vi "LPT-GUI-MIC-ver 5F 2.0.vi"() -> ()   [LabVIEW 2019]
uses:
  <vilib>/userDefined/High Color/IMAQdx.ctl
  LPT/LabView - DISB Eval SW 2.6/LabView - DISB Eval SW 2.6/Register name.ctl
  LPT/LPT-GUI-MIC-ver 5c GLOBAL 1.0.vi
  <vilib>/Utility/file.llb/Write Delimited Spreadsheet (DBL).vi
  <vilib>/vision/driver/NI_Vision_Acquisition_Software.lvlib
panel:
  out "Numeric 9":dbl
  out "Numeric 8":i32
  out "Numeric 7":i32
  out "Numeric 6":i32
  out "Numeric 5":i32
  out "Numeric 4":i32
  out "Numeric 3":i32
  out "Numeric 2":i32
  out "Numeric":i32
  in  "SHUTDOWN\nPROGRAM":bool
  in  "LASER\nOFF":bool
  out "EPOS 1":string
  in  "ACT":refnum<visa-resource-name>="COM5"
  in  "RAMAN Spectometer\n Parameters":T1={"Integration Time (ms)"=80, "Digitizer Clock Rate Setting"=3, "Number of Scans to Average"=1, "Optical Smoothing Level"=0, "C1"=0.096038248763, "C2"=3.43035e-07, "C3"=536.3, "C4"=-1.607e-09, 12}
  in  "LED":refnum<visa-resource-name>="COM5"
  in  "Session In 2":T2="cam6"
  in  "Session In":T2="cam5"
  out "COMMAND1 READ 3":string="LED1 ON\r"
  out "AUT FOCUS STATUS 2":bool
  out "Position (um) 2":dbl(slide) min=0.0 max=100.0 step=0.01 scale=0.0..1500.0
  out "COMMAND 3":string="LED1 OFF"
  out "NUMBER 2":string
  out "Raw Data 2":sgl[](graph)
  out "power sum 2":sgl
  in  "#of steps 3":i32=200
  in  "STAGE START 2":i32
  in  "STAGE STOP 2":i32=20
  out "power sum":sgl
  out "Raw Data":sgl[](graph)
  in  "START CAM TAB":bool
  out "Camera STOP 2":bool
  out "COMMAND1 READ 2":string="LED1 ON\r"
  out "Position (um)":dbl(slide)=1400.0 min=0.0 max=100.0 step=0.01 scale=-10000.0..10000.0
  out "COMMAND 2":string="LED1 OFF"
  out "NUMBER":string
  in  "#of steps 2":i32=5
  in  "STAGE START":i32=-10000
  in  "STAGE STOP":i32=10000
  out "BOROSCOPE END":string
  out "Position (mm)":dbl(slide)=10.0 min=0.0 max=100.0 step=0.01 scale=0.0..20.0 scale format="%.2f"
  out "COMMAND1 READ":string="LED1 ON\r"
  in  "COMMAND 1":string="LED1 OFF"
  out "LASER \nFOCUSED":bool
  in  "INTERACTIVE CONTROLS":T3(radio)
  in  "LQC":refnum<visa-resource-name>="COM4" caption="LQComm resource name"
  in  "ANALYSIS PROGRAM":T4(radio)
  in  "LIBS Laser Frequency (Hz)":u16=10 min=10 max=1000
  in  "Auto Set\nLaser Frequency":bool
  in  "AQUISITION TYPE":enum32{"RAMAN", "LIBS"}(radio)
  in  "Integration\n Time (ms)":i32=100
  in  "ID SPECTRA":bool
  in  "Number of Scans  to Acquire":i32=2
  in  "AutoAcquire":bool=TRUE
  out "power setting from LQ":string="POWER=080\r\n"
  out "Power Out":dbl=0.4
  in  "Get Dark?":bool
  in  "Set Power (mW)":i32=80
  in  "Start":bool
  in  "CAMERA STOP":bool
  in  "EXIT INTERACTIVE\nCONTROL":bool
  in  "ABORT \nLOOP":bool
  out "Removed background":dbl[](graph)
  out "LIBS Dark Spectra":dbl[](graph)
  out "Dark Spectra":dbl[](graph)=[1870.0, 1885.0, 1880.0, 1896.0, 1901.0, 1906.0, 1893.0, 1873.0, 1869.0, 1877.0, 1867.0, 1828.0, 1817.0, 1812.0, 1819.0, 1837.0, 1828.0, 1798.0, 1797.0, 1809.0, 1800.0, 1781.0, 1773.0, 1752.0, 1749.0, 1759.0, 1771.0, 1780.0, 1783.0, 1757.0, 1759.0, 1773.0, 1764.0, 1750.0, 1783.0, 1813.0, 1852.0, 1868.0, 1849.0, 1845.0, 1844.0, 1863.0, 1853.0, 1841.0, 1791.0, 1771.0, 1777.0, 1785.0, 1821.0, 1881.0, 1909.0, 1926.0, 1925.0, 1929.0, 1912.0, 1898.0, 1903.0, 1901.0, 1897.0, 1865.0, 1874.0, 1897.0, 1919.0, 1905.0, 1901.0, 1919.0, 1947.0, 1919.0, 1887.0, 1877.0, 1837.0, 1807.0, 1823.0, 1855.0, 1871.0, 1847.0, 1823.0, 1842.0, 1887.0, 1906.0, 1925.0, 1945.0, 1924.0, 1919.0, 1919.0, 1906.0, 1897.0, 1865.0, 1817.0, 1801.0, 1809.0, 1797.0, 1818.0, 1860.0, 1853.0, 1819.0, 1768.0, 1758.0, 1741.0, 1732.0, 1717.0, 1725.0, 1734.0, 1713.0, 1695.0, 1707.0, 1727.0, 1743.0, 1759.0, 1788.0, 1802.0, 1775.0, 1772.0, 1780.0, 1801.0, 1819.0, 1813.0, 1817.0, 1823.0, 1844.0, 1851.0, 1805.0, 1809.0, 1842.0, 1845.0, 1853.0, 1837.0, 1846.0, 1837.0, 1853.0, 1862.0, 1881.0, 1901.0, 1874.0, 1861.0, 1892.0, 1876.0, 1872.0, 1855.0, 1846.0, 1860.0, 1861.0, 1887.0, 1887.0, 1883.0, 1897.0, 1897.0, 1903.0, 1911.0, 1901.0, 1880.0, 1871.0, 1855.0, 1879.0, 1860.0, 1871.0, 1880.0, 1879.0, 1858.0, 1855.0, 1837.0, 1837.0, 1823.0, 1828.0, 1807.0, 1821.0, 1882.0, 1890.0, 1893.0, 1860.0, 1832.0, 1812.0, 1813.0, 1842.0, 1852.0, 1849.0, 1851.0, 1835.0, 1849.0, 1885.0, 1924.0, 1930.0, 1930.0, 1925.0, 1892.0, 1897.0, 1903.0, 1900.0, 1912.0, 1917.0, 1946.0, 1947.0, 1927.0, 1896.0, 1881.0, 1896.0, 1874.0, 1873.0, 1876.0, 1898.0, 1899.0, 1885.0, 1892.0, 1897.0, 1896.0, 1896.0, 1878.0, 1870.0, 1860.0, 1853.0, 1867.0, 1855.0, 1839.0, 1839.0, 1849.0, 1853.0, 1846.0, 1829.0, 1817.0, 1828.0, 1823.0, 1860.0, 1881.0, 1863.0, 1885.0, 1860.0, 1833.0, 1846.0, 1832.0, 1844.0, 1813.0, 1815.0, 1837.0, 1833.0, 1837.0, 1828.0, 1829.0, 1844.0, 1840.0, 1849.0, 1844.0, 1812.0, 1815.0, 1801.0, 1814.0, 1815.0, 1837.0, 1832.0, 1840.0, 1812.0, 1797.0, 1815.0, 1862.0, 1899.0, 1906.0, 1905.0, 1885.0, 1868.0, 1861.0, 1845.0, 1832.0, 1797.0, 1803.0, 1791.0, 1791.0, 1784.0, 1801.0, 1786.0, 1768.0, 1765.0, 1759.0, 1745.0, 1743.0, 1774.0, 1813.0, 1820.0, 1855.0, 1881.0, 1881.0, 1887.0, 1876.0, 1870.0, 1864.0, 1897.0, 1897.0, 1887.0, 1873.0, 1853.0, 1833.0, 1807.0, 1802.0, 1791.0, 1823.0, 1828.0, 1812.0, 1850.0, 1853.0, 1846.0, 1839.0, 1837.0, 1852.0, 1849.0, 1828.0, 1848.0, 1864.0, 1860.0, 1864.0, 1846.0, 1829.0, 1837.0, 1835.0, 1819.0, 1807.0, 1812.0, 1805.0, 1789.0, 1798.0, 1802.0, 1818.0, 1783.0, 1796.0, 1804.0, 1837.0, 1876.0, 1935.0, 1994.0, 2007.0, 1969.0, 1961.0, 1938.0, 1917.0, 1908.0, 1901.0, 1885.0, 1911.0, 1930.0, 1929.0, 1945.0, 1919.0, 1899.0, 1870.0, 1855.0, 1825.0, 1814.0, 1817.0, 1797.0, 1803.0, 1791.0, 1789.0, 1768.0, 1734.0, 1757.0, 1757.0, 1737.0, 1752.0, 1773.0, 1768.0, 1761.0, 1759.0, 1784.0, 1783.0, 1803.0, 1791.0, 1791.0, 1796.0, 1791.0, 1781.0, 1773.0, 1761.0, 1780.0, 1791.0, 1780.0, 1773.0, 1759.0, 1757.0, 1769.0, 1773.0, 1768.0, 1780.0, 1780.0, 1782.0, 1807.0, 1805.0, 1789.0, 1807.0, 1836.0, 1823.0, 1839.0, 1873.0, 1873.0, 1893.0, 1892.0, 1868.0, 1876.0, 1887.0, 1896.0, 1899.0, 1892.0, 1867.0, 1851.0, 1848.0, 1839.0, 1865.0, 1866.0, 1849.0, 1834.0, 1839.0, 1862.0, 1861.0, 1851.0, 1839.0, 1849.0, 1847.0, 1828.0, 1789.0, 1769.0, 1787.0, 1779.0, 1797.0, 1816.0, 1846.0, 1855.0, 1855.0, 1863.0, 1869.0, 1885.0, 1892.0, 1901.0, 1946.0, 1913.0, 1880.0, 1896.0, 1901.0, 1877.0, 1881.0, 1878.0, 1855.0, 1845.0, 1832.0, 1799.0, 1769.0, 1757.0, 1781.0, 1762.0, 1735.0, 1714.0, 1733.0, 1757.0, 1773.0, 1773.0, 1783.0, 1778.0, 1768.0, 1764.0, 1765.0, 1753.0, 1738.0, 1759.0, 1781.0, 1789.0, 1800.0, 1799.0, 1796.0, 1785.0, 1771.0, 1727.0, 1700.0, 1723.0, 1711.0, 1716.0, 1738.0, 1773.0, 1781.0, 1769.0, 1778.0, 1768.0, 1771.0, 1775.0, 1781.0, 1768.0, 1744.0, 1739.0, 1732.0, 1716.0, 1695.0, 1689.0, 1695.0, 1679.0, 1695.0, 1692.0, 1717.0, 1718.0, 1721.0, 1695.0, 1679.0, 1677.0, 1675.0, 1678.0, 1679.0, 1682.0, 1689.0, 1684.0, 1711.0, 1711.0, 1721.0, 1727.0, 1727.0, 1723.0, 1707.0, 1732.0, 1721.0, 1724.0, 1700.0, 1692.0, 1685.0, 1693.0, 1695.0, 1705.0, 1694.0, 1700.0, 1722.0, 1714.0, 1719.0, 1723.0, 1711.0, 1721.0, 1746.0, 1775.0, 1756.0, 1704.0, 1692.0, 1721.0, 1725.0, 1718.0, 1712.0, 1725.0, 1732.0, 1741.0, 1745.0, 1773.0, 1784.0, 1782.0, 1785.0, 1800.0, 1800.0, 1785.0, 1757.0, 1759.0, 1718.0, 1725.0, 1725.0, 1736.0, 1770.0, 1802.0, 1808.0, 1801.0, 1809.0, 1812.0, 1794.0, 1823.0, 1842.0, 1839.0, 1849.0, 1823.0, 1832.0, 1823.0, 1801.0, 1812.0, 1832.0, 1823.0, 1810.0, 1810.0, 1796.0, 1816.0, 1797.0, 1853.0, 1871.0, 1883.0, 1887.0, 1902.0, 1884.0, 1869.0, 1853.0, 1832.0, 1823.0, 1812.0, 1821.0, 1823.0, 1832.0, 1821.0, 1823.0, 1809.0, 1784.0, 1752.0, 1732.0, 1727.0, 1721.0, 1709.0, 1735.0, 1727.0, 1725.0, 1707.0, 1698.0, 1682.0, 1689.0, 1714.0, 1716.0, 1707.0, 1709.0, 1714.0, 1725.0, 1727.0, 1738.0, 1725.0, 1741.0, 1739.0, 1701.0, 1733.0, 1727.0, 1717.0, 1718.0, 1752.0, 1775.0, 1775.0, 1784.0, 1802.0, 1771.0, 1759.0, 1750.0, 1724.0, 1721.0, 1711.0, 1689.0, 1677.0, 1666.0, 1686.0, 1698.0, 1711.0, 1750.0, 1741.0, 1756.0, 1771.0, 1768.0, 1787.0, 1796.0, 1807.0, 1790.0, 1809.0, 1842.0, 1832.0, 1807.0, 1805.0, 1805.0, 1764.0, 1789.0, 1785.0, 1669.0, 1625.0, 1631.0, 1637.0, 1642.0, 1599.0, 1605.0, 1579.0, 1592.0, 1576.0, 1590.0, 1604.0, 1615.0, 1659.0, 1672.0, 1669.0, 1689.0, 1672.0, 1672.0, 1701.0, 1716.0, 1741.0, 1730.0, 1719.0, 1711.0, 1695.0, 1706.0, 1721.0, 1770.0, 1796.0, 1797.0, 1768.0, 1765.0, 1781.0, 1765.0, 1759.0, 1749.0, 1781.0, 1786.0, 1804.0, 1796.0, 1777.0, 1768.0, 1772.0, 1778.0, 1821.0, 1821.0, 1823.0, 1837.0, 1845.0, 1829.0, 1849.0, 1833.0, 1832.0, 1797.0, 1771.0, 1764.0, 1791.0, 1786.0, 1764.0, 1743.0, 1730.0, 1752.0, 1746.0, 1741.0, 1741.0, 1748.0, 1757.0, 1784.0, 1775.0, 1777.0, 1796.0, 1810.0, 1799.0, 1814.0, 1768.0, 1773.0, 1780.0, 1765.0, 1764.0, 1769.0, 1748.0, 1732.0, 1709.0, 1706.0, 1695.0, 1679.0, 1675.0, 1669.0, 1679.0, 1707.0, 1721.0, 1711.0, 1704.0, 1701.0, 1700.0, 1695.0, 1695.0, 1668.0, 1692.0, 1711.0, 1725.0, 1716.0, 1693.0, 1700.0, 1720.0, 1704.0, 1711.0, 1716.0, 1725.0, 1721.0, 1706.0, 1700.0, 1706.0, 1717.0, 1732.0, 1717.0, 1721.0, 1695.0, 1695.0, 1698.0, 1688.0, 1689.0, 1691.0, 1687.0, 1709.0, 1717.0, 1732.0, 1725.0, 1668.0, 1672.0, 1673.0, 1681.0, 1688.0, 1707.0, 1725.0, 1739.0, 1716.0, 1641.0, 1636.0, 1642.0, 1655.0, 1663.0, 1675.0, 1675.0, 1700.0, 1730.0, 1764.0, 1803.0, 1816.0, 1820.0, 1807.0, 1791.0, 1759.0, 1753.0, 1761.0, 1759.0, 1753.0, 1744.0, 1775.0, 1781.0, 1768.0, 1753.0, 1741.0, 1721.0, 1725.0, 1743.0, 1748.0, 1747.0, 1771.0, 1775.0, 1771.0, 1756.0, 1753.0, 1709.0, 1716.0, 1704.0, 1734.0, 1737.0, 1725.0, 1721.0, 1724.0, 1716.0, 1732.0, 1744.0, 1775.0, 1751.0, 1706.0, 1704.0, 1716.0, 1709.0, 1717.0, 1741.0, 1761.0, 1764.0, 1781.0, 1791.0, 1764.0, 1746.0, 1732.0, 1734.0, 1727.0, 1716.0, 1700.0, 1686.0, 1684.0, 1686.0, 1707.0, 1732.0, 1727.0, 1738.0, 1716.0, 1705.0, 1709.0, 1707.0, 1700.0, 1698.0, 1698.0, 1716.0, 1723.0, 1705.0, 1717.0, 1689.0, 1690.0, 1687.0, 1684.0, 1719.0, 1717.0, 1714.0, 1690.0, 1668.0, 1663.0, 1675.0, 1677.0, 1684.0, 1673.0, 1668.0, 1679.0, 1695.0, 1706.0, 1735.0, 1748.0, 1747.0, 1759.0, 1764.0, 1757.0, 1732.0, 1750.0, 1781.0, 1764.0, 1764.0, 1749.0, 1754.0, 1756.0, 1741.0, 1739.0, 1741.0, 1714.0, 1733.0, 1762.0, 1759.0, 1768.0, 1775.0, 1768.0, 1759.0, 1768.0, 1750.0, 1739.0, 1757.0, 1757.0, 1727.0, 1748.0, 1723.0, 1725.0, 1709.0, 1709.0, 1709.0, 1731.0, 1734.0, 1748.0, 1759.0, 1757.0, 1759.0, 1752.0, 1741.0, 1755.0, 1787.0, 1791.0, 1820.0, 1840.0, 1860.0, 1873.0, 1874.0, 1865.0, 1876.0, 1876.0, 1844.0, 1844.0, 1849.0, 1862.0, 1832.0, 1828.0, 1842.0, 1832.0, 1796.0, 1788.0, 1751.0, 1764.0, 1756.0, 1746.0, 1739.0, 1733.0, 1726.0, 1705.0, 1700.0, 1723.0, 1725.0, 1725.0, 1739.0, 1759.0, 1777.0, 1771.0, 1759.0, 1771.0, 1765.0, 1753.0, 1725.0, 1684.0, 1647.0, 1636.0, 1652.0, 1657.0, 1669.0, 1672.0, 1677.0, 1653.0, 1672.0, 1657.0, 1661.0, 1660.0, 1676.0, 1704.0, 1707.0, 1729.0, 1757.0, 1796.0, 1797.0, 1802.0, 1797.0, 1807.0, 1844.0, 1835.0, 1794.0, 1791.0, 1796.0, 1801.0, 1789.0, 1791.0, 1782.0, 1768.0, 1739.0, 1723.0, 1736.0, 1732.0, 1737.0, 1733.0, 1727.0, 1707.0, 1677.0, 1695.0, 1704.0, 1714.0, 1690.0, 1657.0, 1661.0, 1669.0, 1656.0, 1652.0, 1611.0, 1595.0, 1549.0, 1562.0, 1596.0, 1610.0, 1573.0, 1576.0, 1577.0, 1567.0, 1573.0, 1605.0, 1592.0, 1622.0, 1621.0, 1609.0, 1599.0, 1606.0, 1581.0, 1565.0, 1567.0, 1589.0, 1610.0, 1607.0, 1608.0, 1643.0, 1647.0, 1668.0, 1691.0, 1675.0, 1641.0, 1647.0, 1640.0, 1622.0, 1621.0, 1588.0, 1602.0, 1622.0, 1611.0, 1599.0, 1602.0, 1640.0, 1643.0, 1647.0, 1629.0, 1577.0, 1547.0, 1554.0, 1551.0, 1540.0, 1561.0, 1561.0, 1576.0, 1614.0, 1674.0, 1707.0, 1717.0, 1736.0, 1735.0, 1743.0, 1738.0, 1727.0, 1735.0, 1721.0, 1721.0, 1687.0, 1707.0, 1709.0, 1748.0, 1743.0, 1743.0, 1753.0, 1769.0, 1759.0, 1765.0, 1737.0, 1727.0, 1711.0, 1679.0, 1672.0, 1686.0, 1672.0, 1668.0, 1660.0, 1645.0, 1669.0, 1688.0, 1685.0, 1679.0, 1721.0, 1739.0, 1712.0, 1681.0, 1650.0, 1653.0, 1661.0, 1663.0, 1663.0, 1668.0, 1672.0, 1704.0, 1714.0, 1721.0, 1718.0, 1814.0, 1797.0, 1759.0, 1754.0, 1743.0, 1762.0, 1748.0, 1768.0, 1741.0, 1690.0, 1707.0, 1717.0, 1739.0, 1768.0, 1727.0, 1682.0, 1650.0, 1681.0, 1701.0, 1727.0, 1695.0, 1676.0, 1673.0, 1669.0, 1677.0, 1663.0, 1674.0, 1690.0, 1687.0, 1668.0, 1690.0, 1725.0, 1689.0, 1647.0, 1627.0, 1615.0, 1647.0, 1656.0, 1631.0, 1625.0, 1618.0, 1609.0, 1608.0, 1636.0, 1674.0, 1720.0, 1738.0, 1745.0, 1736.0, 1738.0, 1762.0, 1781.0, 1776.0, 1794.0, 1798.0, 1757.0, 1741.0, 1717.0, 1711.0, 1725.0, 1727.0, 1732.0, 1730.0, 1701.0, 1700.0, 1657.0, 1652.0, 1668.0, 1653.0, 1621.0, 1629.0, 1611.0, 1615.0, 1608.0, 1583.0, 1599.0, 1636.0, 1668.0, 1684.0, 1705.0, 1701.0, 1725.0, 1752.0, 1746.0, 1749.0, 1727.0, 1755.0, 1746.0, 1749.0, 1764.0, 1752.0, 1739.0, 1768.0, 1757.0, 1711.0, 1677.0, 1657.0, 1653.0, 1661.0, 1647.0, 1618.0, 1620.0, 1649.0, 1675.0, 1668.0, 1672.0, 1679.0, 1656.0, 1669.0, 1674.0, 1700.0, 1705.0, 1704.0, 1700.0, 1705.0, 1718.0, 1711.0, 1705.0, 1701.0, 1718.0, 1713.0, 1736.0, 1752.0, 1748.0, 1732.0, 1750.0, 1765.0, 1741.0, 1723.0, 1725.0, 1705.0, 1676.0, 1641.0, 1636.0, 1631.0, 1631.0, 1656.0, 1663.0, 1666.0, 1668.0, 1669.0, 1629.0, 1647.0, 1610.0, 1551.0, 1494.0, 1483.0, 1465.0, 1476.0, 1487.0, 1512.0, 1553.0, 1573.0, 1556.0, 1501.0, 1503.0, 1531.0, 1567.0, 1624.0, 1663.0, 1661.0, 1657.0, 1645.0, 1616.0, 1621.0, 1594.0, 1529.0, 1503.0, 1490.0, 1476.0, 1501.0, 1501.0, 1517.0, 1527.0, 1558.0, 1567.0, 1586.0, 1556.0, 1547.0, 1548.0, 1551.0, 1497.0, 1439.0, 1428.0, 1459.0, 1516.0, 1563.0, 1558.0, 1609.0, 1657.0, 1693.0, 1734.0, 1753.0, 1765.0, 1773.0, 1796.0, 1800.0, 1815.0, 1821.0, 1851.0, 1855.0, 1844.0, 1844.0, 1846.0, 1850.0, 1833.0, 1786.0, 1791.0, 1791.0, 1789.0, 1798.0, 1797.0, 1802.0, 1809.0, 1819.0, 1820.0, 1816.0, 1796.0, 1804.0, 1804.0, 1786.0, 1794.0, 1753.0, 1764.0, 1800.0, 1811.0, 1809.0, 1816.0, 1785.0, 1765.0, 1735.0, 1687.0, 1672.0, 1661.0, 1621.0, 1583.0, 1482.0, 1444.0, 1451.0, 1471.0, 1500.0, 1541.0, 1530.0, 1541.0, 1540.0, 1581.0, 1605.0, 1649.0, 1659.0, 1660.0, 1654.0, 1672.0, 1668.0, 1691.0, 1692.0, 1693.0, 1672.0, 1674.0, 1693.0, 1707.0, 1735.0, 1759.0, 1758.0, 1752.0, 1759.0, 1763.0, 1764.0, 1757.0, 1741.0, 1727.0, 1727.0, 1720.0, 1738.0, 1733.0, 1735.0, 1725.0, 1743.0, 1746.0, 1753.0, 1752.0, 1750.0, 1738.0, 1755.0, 1746.0, 1764.0, 1787.0, 1775.0, 1748.0, 1725.0, 1725.0, 1759.0, 1775.0, 1791.0, 1804.0, 1823.0, 1842.0, 1839.0, 1846.0, 1807.0, 1812.0, 1835.0, 1819.0, 1837.0, 1799.0, 1769.0, 1765.0, 1759.0, 1781.0, 1768.0, 1727.0, 1689.0, 1672.0, 1636.0, 1629.0, 1629.0, 1647.0, 1645.0, 1641.0, 1640.0, 1658.0, 1640.0, 1642.0, 1645.0, 1672.0, 1700.0, 1701.0, 1688.0, 1709.0, 1727.0, 1732.0, 1759.0, 1754.0, 1765.0, 1746.0, 1727.0, 1725.0, 1759.0, 1752.0, 1753.0, 1768.0, 1759.0, 1764.0, 1759.0, 1773.0, 1794.0, 1796.0, 1791.0, 1812.0, 1805.0, 1810.0, 1801.0, 1791.0, 1782.0, 1787.0, 1775.0, 1775.0, 1775.0, 1780.0, 1783.0, 1807.0, 1815.0, 1821.0, 1800.0, 1823.0, 1819.0, 1801.0, 1779.0, 1773.0, 1780.0, 1788.0, 1804.0, 1800.0, 1789.0, 1757.0, 1743.0, 1727.0, 1721.0, 1732.0, 1720.0, 1681.0, 1681.0, 1701.0, 1684.0, 1650.0, 1645.0, 1656.0, 1684.0, 1686.0, 1677.0, 1691.0, 1685.0, 1700.0, 1721.0, 1741.0, 1758.0, 1749.0, 1733.0, 1695.0, 1701.0, 1687.0, 1712.0, 1721.0, 1738.0, 1759.0, 1796.0, 1823.0, 1849.0, 1860.0, 1868.0, 1855.0, 1848.0, 1855.0, 1844.0, 1809.0, 1810.0, 1832.0, 1807.0, 1800.0, 1829.0, 1837.0, 1823.0, 1805.0, 1828.0, 1848.0, 1855.0, 1838.0, 1807.0, 1804.0, 1802.0, 1806.0, 1823.0, 1807.0, 1807.0, 1816.0, 1844.0, 1862.0, 1879.0, 1882.0, 1877.0, 1875.0, 1897.0, 1855.0, 1837.0, 1835.0, 1817.0, 1810.0, 1789.0, 1751.0, 1741.0, 1723.0, 1722.0, 1718.0, 1752.0, 1773.0, 1768.0, 1781.0, 1739.0, 1709.0, 1693.0, 1709.0, 1722.0, 1727.0, 1724.0, 1749.0, 1725.0, 1748.0, 1758.0, 1769.0, 1778.0, 1771.0, 1770.0, 1745.0, 1736.0, 1771.0, 1768.0, 1748.0, 1756.0, 1773.0, 1748.0, 1754.0, 1772.0, 1804.0, 1803.0, 1805.0, 1768.0, 1750.0, 1764.0, 1741.0, 1748.0, 1727.0, 1707.0, 1707.0, 1737.0, 1721.0, 1717.0, 1722.0, 1720.0, 1734.0, 1750.0, 1725.0, 1725.0, 1736.0, 1691.0, 1681.0, 1689.0, 1677.0, 1675.0, 1707.0, 1712.0, 1704.0, 1684.0, 1679.0, 1677.0, 1683.0, 1663.0, 1636.0, 1640.0, 1640.0, 1657.0, 1669.0, 1677.0, 1704.0, 1727.0, 1769.0, 1741.0, 1749.0, 1759.0, 1757.0, 1762.0, 1750.0, 1749.0, 1759.0, 1759.0, 1775.0, 1773.0, 1823.0, 1815.0, 1807.0, 1821.0, 1813.0, 1805.0, 1817.0, 1813.0, 1821.0, 1807.0, 1803.0, 1805.0, 1821.0, 1828.0, 1817.0, 1805.0, 1802.0, 1791.0, 1776.0, 1768.0, 1770.0, 1755.0, 1738.0, 1764.0, 1757.0, 1751.0, 1759.0, 1762.0, 1786.0, 1771.0, 1775.0, 1801.0, 1807.0, 1797.0, 1786.0, 1855.0, 1879.0, 1878.0, 1852.0, 1834.0, 1845.0, 1849.0, 1869.0, 1865.0, 1855.0, 1885.0, 1885.0, 1860.0, 1812.0, 1803.0, 1790.0, 1784.0, 1773.0, 1769.0, 1751.0, 1739.0, 1721.0, 1749.0, 1738.0, 1742.0, 1743.0, 1718.0, 1687.0, 1685.0, 1700.0, 1724.0, 1753.0, 1746.0, 1745.0, 1781.0, 1810.0, 1812.0, 1823.0, 1805.0, 1821.0, 1820.0, 1790.0, 1780.0, 1791.0, 1798.0, 1804.0, 1837.0, 1869.0, 1871.0, 1884.0, 1887.0, 1887.0, 1906.0, 1906.0, 1917.0, 1897.0, 1870.0, 1892.0, 1885.0, 1866.0, 1855.0, 1861.0, 1840.0, 1849.0, 1860.0, 1853.0, 1823.0, 1832.0, 1855.0, 1853.0, 1853.0, 1836.0, 1832.0, 1829.0, 1835.0, 1819.0, 1805.0, 1797.0, 1770.0, 1768.0, 1769.0, 1796.0, 1759.0, 1766.0, 1780.0, 1822.0, 1839.0, 1876.0, 1892.0, 1878.0, 1865.0, 1846.0, 1844.0, 1817.0, 1828.0, 1821.0, 1807.0, 1801.0, 1771.0, 1807.0, 1783.0, 1789.0, 1778.0, 1787.0, 1780.0, 1765.0, 1768.0, 1773.0, 1777.0, 1773.0, 1775.0, 1781.0, 1771.0, 1777.0, 1789.0, 1802.0, 1818.0, 1823.0, 1805.0, 1804.0, 1801.0, 1802.0, 1828.0, 1791.0, 1784.0, 1765.0, 1756.0, 1748.0, 1727.0, 1712.0, 1714.0, 1749.0, 1775.0, 1789.0, 1780.0, 1781.0, 1756.0, 1755.0, 1759.0, 1771.0, 1759.0, 1755.0, 1748.0, 1748.0, 1743.0, 1708.0, 1707.0, 1704.0, 1672.0, 1650.0, 1631.0, 1650.0, 1652.0, 1652.0, 1660.0, 1669.0, 1685.0, 1713.0, 1711.0, 1692.0, 1734.0, 1753.0, 1753.0, 1759.0, 1727.0, 1736.0, 1771.0, 1786.0, 1789.0, 1764.0, 1732.0, 1736.0, 1737.0, 1736.0, 1736.0, 1761.0, 1768.0, 1759.0, 1768.0, 1748.0, 1716.0, 1723.0, 1733.0, 1725.0, 1727.0, 1738.0, 1727.0, 1732.0, 1735.0, 1756.0, 1791.0, 1791.0, 1796.0, 1832.0, 1865.0, 1885.0, 1884.0, 1885.0, 1873.0, 1878.0, 1855.0, 1821.0, 1812.0, 1819.0, 1823.0, 1809.0, 1816.0, 1813.0, 1808.0, 1803.0, 1807.0, 1795.0, 1805.0, 1823.0, 1821.0, 1839.0, 1844.0, 1861.0, 1861.0, 1892.0, 1913.0, 1919.0, 1885.0, 1885.0, 1885.0, 1869.0, 1861.0, 1871.0, 1885.0, 1930.0, 1929.0, 1883.0, 1887.0, 1877.0, 1865.0, 1855.0, 1851.0, 1835.0, 1821.0, 1808.0, 1759.0, 1773.0, 1783.0, 1773.0, 1786.0, 1781.0, 1768.0, 1776.0, 1757.0, 1785.0, 1802.0, 1797.0, 1796.0, 1805.0, 1808.0, 1800.0, 1798.0, 1821.0, 1832.0, 1799.0, 1795.0, 1800.0, 1813.0, 1823.0, 1842.0, 1887.0, 1909.0, 1909.0, 1908.0, 1893.0, 1865.0, 1855.0, 1832.0, 1828.0, 1805.0, 1819.0, 1832.0, 1818.0, 1820.0, 1805.0, 1784.0, 1780.0, 1785.0, 1783.0, 1789.0, 1752.0, 1740.0, 1711.0, 1721.0, 1736.0, 1732.0, 1727.0, 1738.0, 1756.0, 1804.0, 1817.0, 1832.0, 1846.0, 1853.0, 1833.0, 1817.0, 1807.0, 1776.0, 1775.0, 1757.0, 1750.0, 1745.0, 1771.0, 1778.0, 1800.0, 1805.0, 1781.0, 1797.0, 1796.0, 1789.0, 1778.0, 1759.0, 1744.0, 1751.0, 1755.0, 1762.0, 1737.0, 1725.0, 1746.0, 1769.0, 1809.0, 1815.0, 1813.0, 1786.0, 1769.0, 1768.0, 1770.0, 1764.0, 1765.0, 1768.0, 1755.0, 1736.0, 1759.0, 0.0, 0.0, 0.0, 0.0, 0.0]
  out "Status":string="INITIALIZING LIBS"
  in  "STAGE STOP A":i32=19 min=10 max=19 format="%.2f"
  in  "STAGE START A":i32=1 min=1 max=10 format="%.2f"
  in  "#of steps A":i32=18 min=2 max=100
  in  "AUT FOCUS":bool
  out "Spectrum":cluster{dbl[], "Dark Array":dbl[]}(graph)
  out "msPerClock":dbl
  in  "SPI clock frequency [Hz]":u32
  in  "*Cal coef":dbl[](array[numeric])=[0.0] format="%.7e"
  in  "*Wavelength axis":dbl[](array[numeric]) format="%.7e"
  in  "Pixel axis":u16[](array[numeric])
  out "Dark spectrum":dbl[](array[numeric])
  out "Ref spectrum":dbl[](array[numeric])
  in  "*Production mode":u16 format="%x"
  in  "*Sensor ctrl":u16
  in  "Skipping start read buffer":u16 max=4096
  in  "Skipping end read buffer":u16=17 min=17 max=4096
  in  "*Last pixel of interest":u16=17 min=17 max=4096
  in  "*First pixel of interest":u16 max=4096
  out "*FW - Reserved":u16
  out "*FW - Variant":u16
  out "*FW - Revision":u16
  out "*Spectrometer SN":u16
  out "Average in progress":bool
  in  "*Auto trig":bool=TRUE
  in  "*Averaging in HW":u16=1
  in  "*Data ready threshold":u16=1
  in  "*MPP mode change":u16
  out "Debug":u16
  out "*ADC offset [counts]":u16
  out "*ADC gain [counts]":u16
  out "Trigger delay MSB":u16
  out "Trigger delay LSB":u16
  out "Pixels ready":u16
  out "*Temperature  [counts] \n(12 bit ADC)":dbl
  out "Sensor exp time MSB":u16
  out "Sensor exp time LSB":u16
  out "*Calib data chars":u16
  out "*Pixels per image":u16
  out "*Detector type":u16
  out "*FW version":u16
  out "*HW version":u16
  out "*PCB SN":u16
  in  "Zero Dark LIBS":dbl[](array[numeric])
  in  "Data\\Dark":bool
  out "MaxPosition":dbl=500.0 format="%#_2f"
  out "max value":sgl=3651732.0
  in  "Zero Dark":dbl[](array[numeric])
  in  "Channel Settings":T5(array[cluster])=[{"Integration Time (msec)"=80, "Xtrate"=1, "Averaging"=5, "Smoothing"=4, "C1"=0.0, "C2"=0.0, "C3"=0.0, "C4"=0.0, "Digitizer Bits"=enum."12"}, {"Integration Time (msec)"=80, "Xtrate"=1, "Averaging"=5, "Smoothing"=4, "C1"=0.0, "C2"=0.0, "C3"=0.0, "C4"=0.0, "Digitizer Bits"=enum."12"}, {"Integration Time (msec)"=80, "Xtrate"=1, "Averaging"=5, "Smoothing"=4, "C1"=0.0, "C2"=0.0, "C3"=0.0, "C4"=0.0, "Digitizer Bits"=enum."12"}, {"Integration Time (msec)"=80, "Xtrate"=1, "Averaging"=5, "Smoothing"=4, "C1"=0.0, "C2"=0.0, "C3"=0.0, "C4"=0.0, "Digitizer Bits"=enum."12"}, {"Integration Time (msec)"=80, "Xtrate"=1, "Averaging"=5, "Smoothing"=4, "C1"=0.0, "C2"=0.0, "C3"=0.0, "C4"=0.0, "Digitizer Bits"=enum."12"}, {"Integration Time (msec)"=80, "Xtrate"=1, "Averaging"=5, "Smoothing"=4, "C1"=0.0, "C2"=0.0, "C3"=0.0, "C4"=0.0, "Digitizer Bits"=enum."12"}, {"Integration Time (msec)"=80, "Xtrate"=1, "Averaging"=5, "Smoothing"=4, "C1"=0.0, "C2"=0.0, "C3"=0.0, "C4"=0.0, "Digitizer Bits"=enum."12"}, {"Integration Time (msec)"=80, "Xtrate"=1, "Averaging"=5, "Smoothing"=4, "C1"=0.0, "C2"=0.0, "C3"=0.0, "C4"=0.0, "Digitizer Bits"=enum."12"}] caption="Spectrometer Configs" {"C4" format="%#.15f"; "C3" format="%#.15f"; "C2" format="%#.15f"; "C1" format="%#.15f"; "Smoothing" min=0 max=4 step=1; "Averaging" min=1 max=10000 step=1; "Xtrate" min=1 max=3; "Integration Time (msec)" min=1 max=2000}
  out "output\ncluster":T6={"Integration Time (ms)"=80, "Digitizer Clock Rate Setting"=3, "Number of Scans to Average"=1, "Optical Smoothing Level"=0, 0.096038248763, 3.43035e-07, -1.607e-09, -1.607e-09, 12}
  in  "Tab Control":enum32{"Visible", "Fluorescence"}(tab)
  out "Visible Image":T7(plugin-control)
  out "Fluorescence Image":T7(plugin-control)
  in  "MOVE SPECTROMETER":bool
  out "AUT FOCUS STATUS":bool
  in  "Set End Position (um)":dbl(slide) scale=0.0..1500.0
  out "LED 2 STATUS":bool
  in  "LED 2":bool
  in  "LED 1":bool
  out "LED 1 STATUS":bool
  # "Laser and Plasma RAMAN/LIBS Acquisition Software V5F"
  # "INITIAL SETTINGS"
  # "Raman Laser Settings"
  # "LIBS Laser Settings"
  # "AUTO FOCUS SETTINGS"
  # "AUTO FOCUS RESULTS"
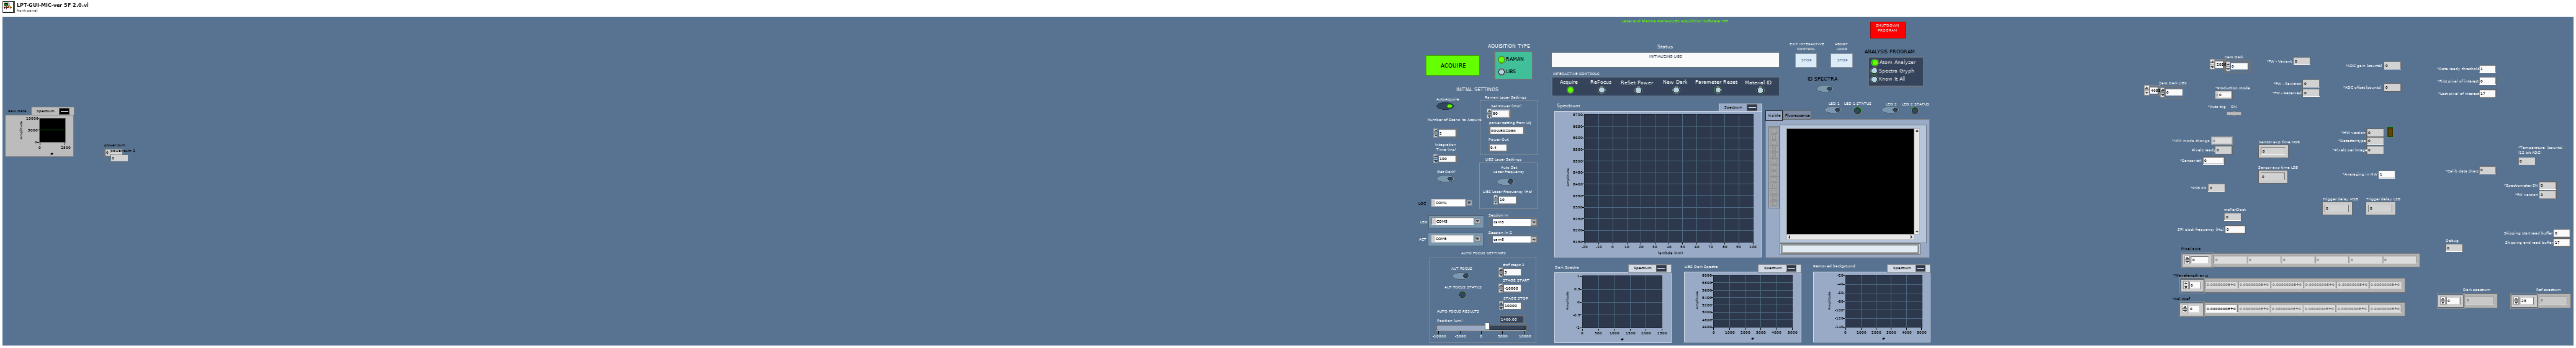
[diagram p1: front panel]
types:
  T1 = typedef "Control 1.ctl" = cluster{"Integration Time (ms)":i32, "Digitizer Clock Rate Setting":i32, "Number of Scans to Average":i32, "Optical Smoothing Level":i32, "C1":dbl, "C2":dbl, "C3":dbl, "C4":dbl, i32}
  T2 = typedef "IMAQdx.ctl" = refnum<k21>
  T3 = enum32{"Acquire", "ReFocus", "ReSet Power", "New Dark", "Parameter Reset", "Material ID", "Do Nothing"}
  T4 = enum32{"Atom Analyzer", "Spectra Gryph", "Know It All"}
  T5 = cluster{"Integration Time (msec)":i32, "Xtrate":i32, "Averaging":i32, "Smoothing":i32, "C1":dbl, "C2":dbl, "C3":dbl, "C4":dbl, "Digitizer Bits":enum8{"12", "14", "16"}}[]
  T6 = cluster{"Integration Time (ms)":i32, "Digitizer Clock Rate Setting":i32, "Number of Scans to Average":i32, "Optical Smoothing Level":i32, dbl, dbl, dbl, dbl, i32}
  T7 = typedef "IMAQ Image.ctl" = refnum<image>
  T8 = typedef "Register name.ctl" = enum8{"Serial number", "HW version", "FW version", "Detector type", "Pixel per image", "Calib data chars", "Calib data", "Sensor ctrl", "Sensor exp time LSB", "Sensor exp time MSB", "Temperature", "Pixel ready", "Trigger delay LSB", "Trigger delay MSB", "ADC PGA", "ADC offset", "Permanent storage", "MPP mode change", "DATA READY THRESHOLD", "IMAGES_TO_AVERAGE", "AVG_CONTROL", "SPECTROMETER SN", "SKIPPING_START", "SKIPPING_END", "debug", "Production mode"}
  T9 = enum8{"Enabled", "Disabled", "Disabled and Grayed Out"}
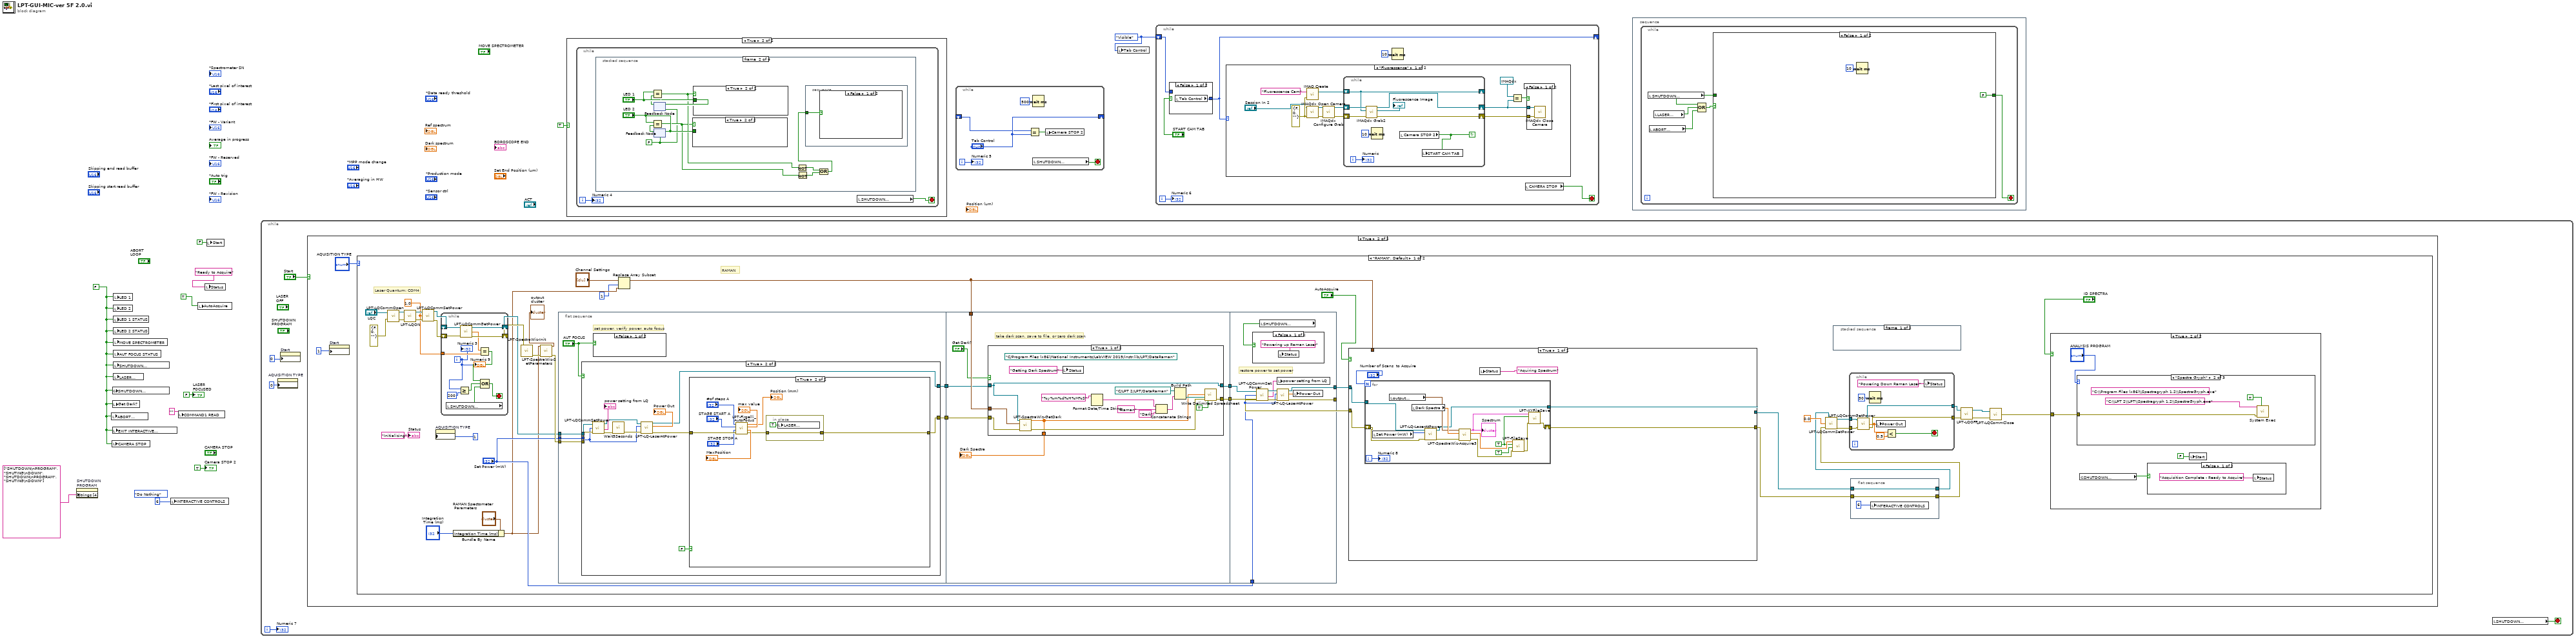
[diagram p0: block diagram]
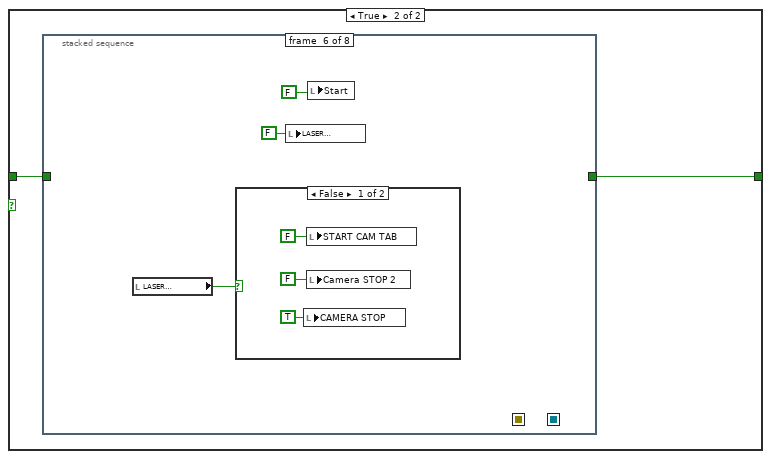
[diagram p2: hidden frame]
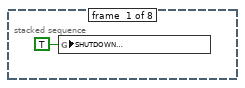
[diagram p3: hidden frame]
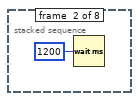
[diagram p4: hidden frame]
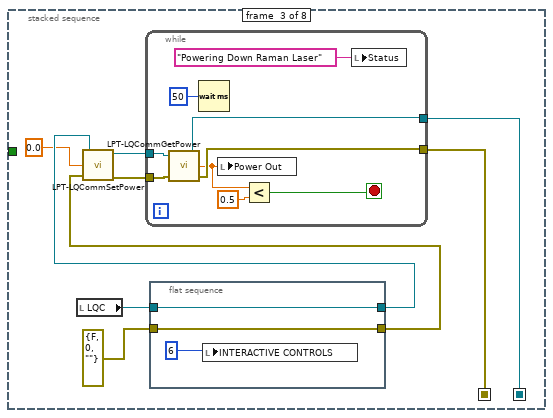
[diagram p5: hidden frame]
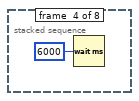
[diagram p6: hidden frame]
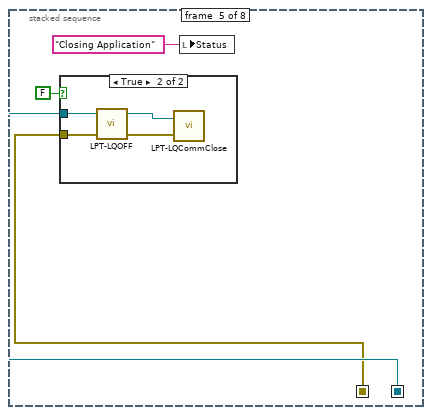
[diagram p7: hidden frame]
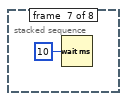
[diagram p10: hidden frame]
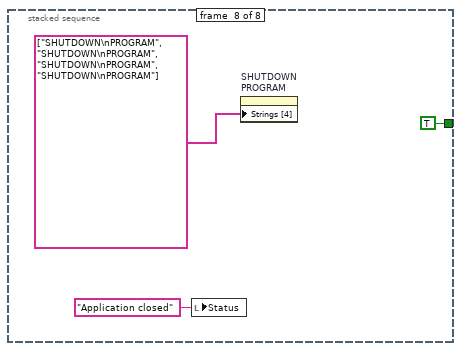
[diagram p11: hidden frame]
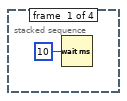
[diagram p13: hidden frame]
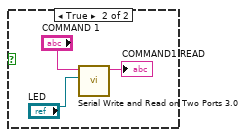
[diagram p14: hidden frame]
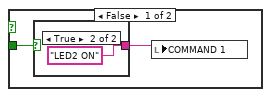
[diagram p15: hidden frame]
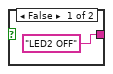
[diagram p16: hidden frame]
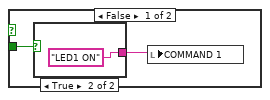
[diagram p17: hidden frame]
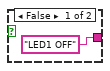
[diagram p18: hidden frame]
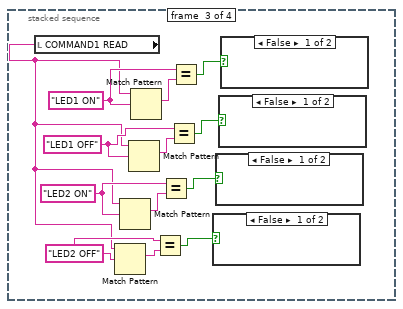
[diagram p19: hidden frame]
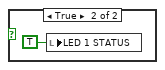
[diagram p20: hidden frame]
diagram:
  (unwired) T3."Do Nothing" ("INTERACTIVE CONTROLS")
  w5 = enum32{"Visible", "Fluorescence"}."Visible" ("Tab Control")
  w2 = FALSE
  n1 = property on="SHUTDOWN\nPROGRAM" class="Bool (strict)"("Strings [4]"=string[] ["SHUTDOWN\nPROGRAM", "SHUTING\nDOWN", "SHUTDOWN\nPROGRAM", "SHUTING\nDOWN"]) -> ()  [unwired: 2 in, 2 out]
  n2 = local write "ABORT \nLOOP"(w2) -> ()
  n3 = local write "CAMERA STOP"(w2) -> ()
  n4 = global write "LPT-GUI-MIC-ver 5c GLOBAL 1.0.vi" "SHUTDOWN\nPROGRAM"(w2) -> ()
  n5 = local write "Get Dark?"(w2) -> ()
  n6 = local write "EXIT INTERACTIVE\nCONTROL"(w2) -> ()
  n7 = local write "LED 1"(w2) -> ()
  n8 = local write "LED 2"(w2) -> ()
  n9 = local write "LED 1 STATUS"(w2) -> ()
  n10 = local write "LED 2 STATUS"(w2) -> ()
  n11 = local write "MOVE SPECTROMETER"(w2) -> ()
  n12 = local write "AUT FOCUS STATUS"(w2) -> ()
  n13 = local write "SHUTDOWN\nPROGRAM"(w2) -> ()
  n14 = local write "LASER\nOFF"(w2) -> ()
  n15 = local write "INTERACTIVE CONTROLS"(6) -> ()
  n16 = local write "COMMAND1 READ"("" ("COMMAND1 READ")) -> ()
  n17 = local write "AutoAcquire"(TRUE ("AutoAcquire")) -> ()
  n18 = local write "Status"("Ready to Acquire") -> ()
  n19 = local write "Start"(FALSE) -> ()
  n20 = while {
    i -> [w12]
    stop <- w13 stop-if-true
    n21 = property on="AQUISITION TYPE" class="RadioBtnsControl (strict)"("DisabledEnum"=0) -> ()  [unwired: 2 in, 2 out]
    n22 = property on="Start" class="Bool (strict)"("DisabledEnum"=0) -> ()  [unwired: 2 in, 2 out]
    n23 = case shown="True" "Start" {
      frame False {
      }
      frame True {
        n24 = property on="Start" class="Bool (strict)"("DisabledEnum"=1) -> ()  [unwired: 2 in, 2 out]
        n25 = case shown="\"RAMAN\", Default" "AQUISITION TYPE" {
          frame "RAMAN", Default {
            w41 = 1.0 ("Set Power (mW)")
            # "RAMAN"
            # "Laser Quantum: COM4"
            n26 = call "LPT-LQCommOpen.vi"("error in"=errorcluster {"status"=FALSE, "code"=0, "source"=""}, "LQComm resource name"="LQC") -> ("error out"=w55:errorcluster, "LQComm Resource out"=w56:refnum<visa-resource-name>)
            n27 = call "LPT-LQON.vi"("error in"=w55, "LQComm Resource In"=w56) -> ("error out"=w45:errorcluster, "LQComm Resource Out"=w44:refnum<visa-resource-name>)  [unwired: 1 in, 1 out]
            n28 = call "LPT-LQCommSetPower.vi"("LQComm Resource In"=w44, "Set Power (mW)"=w41, "error in"=w45) -> ("LQComm Resource Out"=w43:refnum<visa-resource-name>, "error out"=w42:errorcluster)  [unwired: 2 out]
            n29 = property on="AQUISITION TYPE" class="RadioBtnsControl (strict)"("DisabledEnum"=1) -> ()  [unwired: 2 in, 2 out]
            n30 = while {
              shift-right: [w83] -> w39
              shift-left: w43 -> [w85]
              shift-right: [w84] -> w40
              shift-left: w42 -> [w82]
              tunnel: w41 -> [w80]
              i -> [w77]
              stop <- w78 stop-if-true
              n31 = local read "SHUTDOWN\nPROGRAM"() -> (w75:bool)
              n32 = Greater Or Equal?(x=w77, y=200) -> (x >= y?=w74:bool)
              n33 = call "LPT-LQCommGetPower.vi"("error in"=w82, "LQComm Resource In"=w85) -> ("error out"=w84:errorcluster, "NumericValue"=w81:dbl, "LQComm Resource Out"=w83:refnum<visa-resource-name>)  [unwired: 1 in]
              n34 = Equal?(x=w81, y=w80) -> (x = y?=w79:bool)
              n35 = Compound Arithmetic op=OR(w79, w74, w75) -> (w78:bool)
              "Numeric 3" <- w77
              "Numeric 9" <- w77
            }
            n36 = Bundle By Name(cluster="RAMAN Spectometer\n Parameters", "Integration Time (ms)"="Integration\n Time (ms)") -> (w36:T1)
            n37 = call "LPT-SpectraWiz-Init.vi"("error in (no error)"=w40) -> ("error out"=w53:errorcluster)  [unwired: 10 in]
            n38 = call "LPT-SpectraWiz-SetParameters.vi"("error in"=w53, "input cluster"=w36) -> ("error out"=w52:errorcluster, "output cluster"=→"output\ncluster":T6)  [unwired: 8 in]
            n39 = flat-sequence {
              tunnel: w52 -> [w245]
              tunnel: "Set Power (mW)" -> [w246]
              tunnel: [w244] -> w61
              tunnel: [w243] -> w60
              tunnel: w39 -> [w242]
              tunnel: w29 -> [w331]
              tunnel: [w330] -> w59
              tunnel: w61 -> [w328]
              tunnel: w60 -> [w326]
              tunnel: [w327] -> w58
              tunnel: "Set Power (mW)" -> [w357]
              tunnel: w59 -> [w360]
              tunnel: [w356] -> w50
              tunnel: w58 -> [w355]
              tunnel: [w354] -> w49
              frame #0 {
                # "set power, verify power, auto focus"
                n40 = case shown="True" "AUT FOCUS" {
                  tunnel: w246 -> [_ w255]
                  tunnel: w245 -> [w249 w260]
                  tunnel: [w249 w252] -> w244
                  tunnel: [w248 w250] -> w243
                  tunnel: w242 -> [w248 w256]
                  frame False {
                  }
                  frame True {
                    n41 = call "LPT-LQCommSetPower.vi"("LQComm Resource In"=w256, "Set Power (mW)"=w255, "error in"=w260) -> ("LQComm Resource Out"=w259:refnum<visa-resource-name>, "decimal integer string"=→"power setting from LQ":string, "error out"=w258:errorcluster)  [unwired: 1 out]
                    n42 = call "Wait5Seconds.vi"("error in"=w258) -> ("error out"=w257:errorcluster)  [unwired: 10 in]
                    n43 = call "LPT-LQ-LaserAtPower.vi"("error in"=w257, "Set Power (mW)"=w255, "LQComm Resource In"=w259) -> ("error out"=w253:errorcluster, "Power Out"=→"Power Out":dbl, "LQComm Resource Out"=w250:refnum<visa-resource-name>)  [unwired: 5 in, 1 out]
                    n44 = case shown="True" FALSE {
                      tunnel: w253 -> [w262 w320]
                      tunnel: [w263 w315] -> w252
                      frame False {
                        n45 = stacked-sequence {
                          seq-local: [w266 _ _] -> [_ w303 _]
                          seq-local: [w265 _ _] -> [_ w306 _]
                          seq-local: ["STAGE START" _ _] -> [_ w307 _]
                          tunnel: [w268 _ _] -> w263
                          tunnel: w262 -> [w268 _ _]
                          frame #0 {
                            n46 = Subtract(x="STAGE STOP", y="STAGE START") -> (x-y=w270:i32)
                            n47 = Divide(x=w270, y="#of steps 2") -> (x/y=w265:dbl)
                            n48 = Increment(x="#of steps 2") -> (x+1=w271:i32)
                            n49 = for {
                              N: w271 -> [_]
                              tunnel: w265 -> [w281]
                              tunnel: "STAGE START" -> [w277]
                              shift-right: [w273] -> w266
                              shift-left: sgl[] [] -> [w274]
                              i -> [w280]
                              n50 = stacked-sequence {
                                tunnel: [_ w283] -> w275
                                frame #0 {
                                n51 = Wait (ms)(milliseconds to wait=u32 1000) -> ()  [unwired: 1 out]
                                }
                                frame #1 {
                                n52 = call "LPT-SpectraWiz-Acquire W Dark.vi"() -> ("Buffer"=w283:sgl[])  [unwired: 10 in, 1 out]
                                }
                              }
                              "Raw Data" <- w275
                              n53 = Multiply(x=w281, y=w280) -> (x*y=w279:dbl)
                              n54 = Add(x=w277, y=w279) -> (x+y=w278:dbl)
                              n55 = stacked-sequence {
                                tunnel: w278 -> [_ w289 _ _ _]
                                frame #0 {
                                n56 = local write "AUT FOCUS STATUS"(FALSE ("AUT FOCUS STATUS")) -> ()
                                }
                                frame #1 {
                                # "MOV"
                                n57 = Number To Decimal String(number=w289) -> (decimal integer string=w287:string)  [unwired: 1 in]
                                n58 = Concatenate Strings("DPOS=", w287) -> (→"COMMAND 2":string)
                                n59 = Concatenate Strings("DPOS=", w287) -> (→"NUMBER":string)
                                }
                                frame #2 {
                                n60 = local read "COMMAND 2"() -> (w293:string)
                                n61 = local read "NUMBER"() -> (w295:string)
                                n62 = local read "ACT"() -> (w292:refnum<visa-resource-name>)
                                n63 = call "Serial Write and Read on Two Ports 4.0.vi"("VISA Resource (write)"=w292, "Write String"=w293) -> ("Read String"=w291:string)  [unwired: 9 in]
                                "COMMAND1 READ 2" <- w291
                                "EPOS 1" <- w291
                                n64 = Match Pattern(string=w291, regular expression=w295) -> ()  [unwired: 1 in, 4 out]
                                n65 = Equal?(x=w291, y=w291) -> (x = y?=→"AUT FOCUS STATUS":bool)
                                }
                                frame #3 {
                                n66 = local read "COMMAND1 READ 2"() -> (w301:string)
                                n67 = Match Pattern(string=w301, regular expression="EPOS=") -> (after substring=w299:string)  [unwired: 1 in, 3 out]
                                n68 = Match Pattern(string=w299, regular expression="\\n") -> (before substring=w297:string)  [unwired: 1 in, 3 out]
                                n69 = Decimal String To Number(string=w297) -> (number=w296:i32)  [unwired: 2 in, 1 out]
                                n70 = local write "Position (um)"(w296) -> ()
                                }
                                frame #4 {
                                n71 = Wait (ms)(milliseconds to wait=u32 100) -> ()  [unwired: 1 out]
                                }
                              }
                              n72 = Add Array Elements(numeric array=w275) -> (sum=w276:sgl)
                              "power sum" <- w276
                              n73 = Build Array (concatenate)(w274, w276) -> (w273:sgl[])
                            }
                          }
                          frame #1 {
                            (unwired) 10.0 ("Position (mm)")
                            (unwired) 500.0 ("MaxPosition")
                            (unwired) sgl 3651732.0 ("max value")
                            n74 = Array Max & Min(array=w303) -> (max value=w305:sgl, max index (indices)=w309:i32)  [unwired: 2 out]
                            n75 = Multiply(x=w309, y=w306) -> (x*y=w308:dbl)
                            n76 = local write "max value"(w305) -> ()
                            n77 = Add(x=w308, y=w307) -> (x+y=w304:dbl)
                            n78 = local write "MaxPosition"(w304) -> ()
                            n79 = local write "Position (um)"(w304) -> ()
                          }
                          frame #2 {
                            n80 = local read "Position (um)"() -> (w311:dbl)
                            n81 = Number To Decimal String(number=w311) -> (decimal integer string=w312:string)  [unwired: 1 in]
                            n82 = Concatenate Strings("DPOS=", w312) -> (w310:string)
                            n83 = call "Serial Write and Read on Two Ports 4.0.vi"("Write String"=w310) -> ()  [unwired: 10 in, 1 out]
                          }
                        }
                      }
                      frame True {
                        n84 = call "LPT-Firgelli_AutoFocus.vi"("error in (no error)"=w320, "STOP"="STAGE STOP A", "START"="STAGE START A", "#of steps"="#of steps A") -> ("error out"=w316:errorcluster, "MaxPosition"=→"MaxPosition":dbl, "max value"=→"max value":sgl, "Position (mm)"=→"Position (mm)":dbl)  [unwired: 3 in, 1 out]
                        n85 = in-place {
                          in-place-border: w316 -> [w324]
                          in-place-border: [w324] -> w315
                          n86 = local write "LASER \nFOCUSED"(TRUE ("Laser \nFocused")) -> ()
                        }
                      }
                    }
                  }
                }
                n87 = case shown="False" "AUT FOCUS" {
                  frame False {
                  }
                  frame True {
                    n88 = local write "Status"("Autofocus") -> ()
                  }
                }
              }
              frame #1 {
                # "take dark scan, save to file, or zero dark scan"
                n89 = case shown="True" "Get Dark?" {
                  tunnel: w331 -> [w346 _]
                  tunnel: [w343 w349] -> w330
                  tunnel: [w334 "Zero Dark"] -> w329
                  tunnel: w328 -> [w336 w350]
                  tunnel: w326 -> [w335 w352]
                  tunnel: [w335 w352] -> w327
                  frame True {
                    (unwired) path "C:/Program Files (x86)/National Instruments/LabVIEW 2019/instr.lib/LPT/DataRaman" ("base path")
                    n90 = call "LPT-SpectraWiz-GetDark.vi"("error in"=w336, "Channel Settings"=w346, "LQComm Resource In"=w335) -> ("error out"=w344:errorcluster, "Dark Spectra"=w334:sgl[])  [unwired: 7 in]
                    n91 = local write "Status"("Getting Dark Spectrum") -> ()
                    n92 = Format Date/Time String(time format string (%c)="%y%m%d%H%M%S") -> (date/time string=w340:string)  [unwired: 2 in]
                    n93 = Concatenate Strings(w340, "Raman" ("string"), "Dark" ("string")) -> (w342:string)
                    n94 = Build Path(base path=path "C:/LPT 2/LPT/DataRaman", name or relative path=w342) -> (appended path=w345:path)
                    n95 = call-poly <vilib>:"Write Delimited Spreadsheet.vi"("file path (dialog if empty)"=w345, "1D data"=w334, "error in (no error)"=w344, "transpose? (no:F)"=TRUE) -> ("error out"=w343:errorcluster)  [unwired: 10 in, 1 out]
                  }
                  frame False {
                    n96 = local read "Start"() -> (w347:bool)
                    n97 = call "LPT-FileSave.vi"("error in (no error)"=w350, "Data\\Dark"="Data\\Dark", "Raman\\LIBS"=w347, "Array"="Zero Dark") -> ("error out"=w349:errorcluster)  [unwired: 7 in]
                  }
                }
                "Dark Spectra" <- w329
              }
              frame #2 {
                # "restore power to set power"
                n98 = call "LPT-LQCommSetPower.vi"("LQComm Resource In"=w355, "Set Power (mW)"=w357, "error in"=w360) -> ("LQComm Resource Out"=w361:refnum<visa-resource-name>, "decimal integer string"=w358:string, "error out"=w362:errorcluster)  [unwired: 1 out]
                n99 = local read "SHUTDOWN\nPROGRAM"() -> (w353:bool)
                n100 = case shown="False" w353 {
                  frame False {
                    n101 = local write "Status"("Powering up Raman Laser" ("STATUS")) -> ()
                  }
                  frame True {
                  }
                }
                n102 = local write "power setting from LQ"(w358) -> ()
                n103 = call "LPT-LQ-LaserAtPower.vi"("error in"=w362, "Set Power (mW)"=w357, "LQComm Resource In"=w361) -> ("error out"=w356:errorcluster, "Power Out"=w359:dbl, "LQComm Resource Out"=w354:refnum<visa-resource-name>)  [unwired: 5 in, 1 out]
                n104 = local write "Power Out"(w359) -> ()
              }
            }
            n105 = Replace Array Subset(array="Channel Settings", new element=w36, index=u32 1 ("Channel\n(1-based)")) -> (w29:T5)
            n106 = case shown="True" "AutoAcquire" {
              tunnel: [w110 w130] -> w30
              tunnel: w50 -> [w105 w129]
              tunnel: w49 -> [w109 w128]
              tunnel: [w106 w127] -> w28
              tunnel: w29 -> [_ w126]
              frame True {
                n107 = for {
                  N: "Number of Scans  to Acquire" -> [_]
                  tunnel: w109 -> [w124]
                  shift-right: [w113] -> w110
                  shift-left: w105 -> [w125]
                  tunnel: [w112] -> w106
                  i -> [w111]
                  w115 = TRUE ("Raman\\LIBS")
                  n108 = local read "Set Power (mW)"() -> (w122:i32)
                  n109 = local read "output\ncluster"() -> (w117:T6)
                  n110 = local read "Dark Spectra"() -> (w121:dbl[])
                  n111 = call "LPT-LQ-LaserAtPower.vi"("error in"=w125, "Set Power (mW)"=w122, "LQComm Resource In"=w124) -> ("error out"=w123:errorcluster, "LQComm Resource Out"=w112:refnum<visa-resource-name>)  [unwired: 5 in, 2 out]
                  n112 = call "LPT-SpectraWiz-Acquire3.vi"("error in"=w123, "Dark Array"=w121, "input cluster"=w117) -> ("error out"=w119:errorcluster, "Raw Data"=w120:sgl[], "Spectrum"=w116:cluster{dbl[], "Dark Array":dbl[]})  [unwired: 5 in, 1 out]
                  "Spectrum" <- w116
                  n113 = call "LPT-FileSave.vi"("error in (no error)"=w119, "Data\\Dark"=TRUE ("Data\\Dark"), "Raman\\LIBS"=w115, "Array"=w120) -> ("error out"=w114:errorcluster)  [unwired: 7 in]
                  n114 = call "LPT-XYFileSave.vi"("error in (no error)"=w114, "Raman\\LIBS"=w115, "Spectrum"=w116) -> ("error out"=w113:errorcluster)  [unwired: 8 in]
                  "Numeric 8" <- w111
                }
                n115 = local write "Status"("Aquiring Spectrum" ("STATUS")) -> ()
              }
              frame False {
                n116 = while {
                  tunnel: [w133] -> w130
                  tunnel: w129 -> [w135]
                  tunnel: w128 -> [w134]
                  tunnel: [w132] -> w127
                  tunnel: w126 -> [w131]
                  stop <- "EXIT INTERACTIVE\nCONTROL" stop-if-true
                  n117 = case shown="\"Acquire\", Default" "INTERACTIVE CONTROLS" {
                    tunnel: w135 -> [w142 w160 w182 w194 w212 w220 w237]
                    tunnel: w134 -> [w141 w159 w181 w195 w211 w219 w238]
                    tunnel: [w140 w155 w178 w205 w209 w217 w236] -> w133
                    tunnel: [w139 w159 w180 w195 w211 w219 w238] -> w132
                    tunnel: w131 -> [_ _ _ w192 _ _ _]
                    frame "Acquire", Default {
                      n118 = local read "Set Power (mW)"() -> (w146:i32)
                      n119 = local read "Dark Spectra"() -> (w147:dbl[])
                      n120 = call "LPT-LQ-LaserAtPower.vi"("error in"=w142, "Set Power (mW)"=w146, "LQComm Resource In"=w141) -> ("error out"=w145:errorcluster, "LQComm Resource Out"=w139:refnum<visa-resource-name>)  [unwired: 5 in, 2 out]
                      n121 = local read "output\ncluster"() -> (w149:T6)
                      n122 = call "LPT-SpectraWiz-Acquire3.vi"("error in"=w145, "Dark Array"=w147, "input cluster"=w149) -> ("error out"=w148:errorcluster, "Raw Data"=w151:sgl[], "Spectrum"=w150:cluster{dbl[], "Dark Array":dbl[]})  [unwired: 5 in, 1 out]
                      n123 = local write "Spectrum"(w150) -> ()
                      n124 = call "LPT-FileSave.vi"("error in (no error)"=w148, "Data\\Dark"=TRUE ("Data\\Dark"), "Raman\\LIBS"=TRUE ("Raman\\LIBS"), "Array"=w151) -> ("error out"=w152:errorcluster)  [unwired: 7 in]
                      n125 = flat-sequence {
                        tunnel: w152 -> [w153]
                        tunnel: [w153] -> w140
                        frame #0 {
                          n126 = Wait (ms)(milliseconds to wait=1000) -> ()  [unwired: 1 out]
                        }
                      }
                    }
                    frame "ReFocus" {
                      n127 = local read "Set End Position (um)"() -> (w165:dbl)
                      n128 = Less?(x=w165, y=2) -> (x < y?=w164:bool)
                      n129 = case shown="False" w164 {
                        tunnel: w165 -> [w174 _]
                        tunnel: [w172 1] -> w166
                        tunnel: [w171 3] -> w167
                        frame False {
                          n130 = Subtract(x=w174, y=1) -> (x-y=w172:dbl)
                          n131 = Add(x=w172, y=2) -> (x+y=w171:dbl)
                        }
                        frame True {
                        }
                      }
                      n132 = call "LPT-Firgelli_AutoFocus.vi"("error in (no error)"=w160, "STOP"=w167, "START"=w166, "#of steps"=10) -> ("error out"=w156:errorcluster, "MaxPosition"=w163:dbl, "max value"=w162:sgl, "Position (mm)"=w161:dbl)  [unwired: 3 in, 1 out]
                      n133 = local write "Set End Position (um)"(w161) -> ()
                      n134 = local write "max value"(w162) -> ()
                      n135 = local write "MaxPosition"(w163) -> ()
                      n136 = flat-sequence {
                        tunnel: w156 -> [w170]
                        tunnel: [w170] -> w155
                        frame #0 {
                          n137 = local write "INTERACTIVE CONTROLS"(6) -> ()
                          n138 = Wait (ms)(milliseconds to wait=1000) -> ()  [unwired: 1 out]
                        }
                      }
                    }
                    frame "ReSet Power" {
                      n139 = local read "Set Power (mW)"() -> (w185:i32)
                      n140 = call "LPT-LQCommSetPower.vi"("LQComm Resource In"=w181, "Set Power (mW)"=w185, "error in"=w182) -> ("LQComm Resource Out"=w186:refnum<visa-resource-name>, "decimal integer string"=w184:string, "error out"=w187:errorcluster)  [unwired: 1 out]
                      n141 = local write "power setting from LQ"(w184) -> ()
                      n142 = call "LPT-LQ-LaserAtPower.vi"("error in"=w187, "Set Power (mW)"=w185, "LQComm Resource In"=w186) -> ("error out"=w179:errorcluster, "Power Out"=w183:dbl, "LQComm Resource Out"=w180:refnum<visa-resource-name>)  [unwired: 5 in, 1 out]
                      n143 = local write "Power Out"(w183) -> ()
                      n144 = flat-sequence {
                        tunnel: [w190] -> w178
                        tunnel: w179 -> [w190]
                        frame #0 {
                          n145 = local write "INTERACTIVE CONTROLS"(6) -> ()
                          n146 = Wait (ms)(milliseconds to wait=1000) -> ()  [unwired: 1 out]
                        }
                      }
                    }
                    frame "New Dark" {
                      (unwired) path "C:/Program Files (x86)/National Instruments/LabVIEW 2019/instr.lib/LPT/DataRaman" ("base path")
                      n147 = call "LPT-SpectraWiz-GetDark.vi"("error in"=w194, "Channel Settings"=w192, "LQComm Resource In"=w195) -> ("error out"=w203:errorcluster, "Dark Spectra"=w196:sgl[])  [unwired: 7 in]
                      n148 = local write "Dark spectrum"(w196) -> ()
                      n149 = Format Date/Time String(time format string (%c)="%y%m%d%H%M%S") -> (date/time string=w200:string)  [unwired: 2 in]
                      n150 = Concatenate Strings(w200, "Raman" ("string"), "Dark" ("string")) -> (w202:string)
                      n151 = Build Path(base path=path "C:/LPT 2/LPT/DataRaman", name or relative path=w202) -> (appended path=w204:path)
                      n152 = call-poly <vilib>:"Write Delimited Spreadsheet.vi"("file path (dialog if empty)"=w204, "1D data"=w196, "error in (no error)"=w203, "transpose? (no:F)"=TRUE) -> ("error out"=w193:errorcluster)  [unwired: 10 in, 1 out]
                      n153 = flat-sequence {
                        tunnel: w193 -> [w208]
                        tunnel: [w208] -> w205
                        frame #0 {
                          n154 = local write "INTERACTIVE CONTROLS"(6) -> ()
                          n155 = Wait (ms)(milliseconds to wait=1000) -> ()  [unwired: 1 out]
                        }
                      }
                    }
                    frame "Parameter Reset" {
                      n156 = local read "output\ncluster"() -> (w213:T6)
                      n157 = call "LPT-SpectraWiz-SetParameters.vi"("error in"=w212, "input cluster"=w213) -> ("error out"=w210:errorcluster)  [unwired: 8 in, 1 out]
                      n158 = flat-sequence {
                        tunnel: w210 -> [w216]
                        tunnel: [w216] -> w209
                        frame #0 {
                          n159 = local write "INTERACTIVE CONTROLS"(6) -> ()
                          n160 = Wait (ms)(milliseconds to wait=1000) -> ()  [unwired: 1 out]
                        }
                      }
                    }
                    frame "Material ID" {
                      n161 = local read "ANALYSIS PROGRAM"() -> (w221:T4)
                      n162 = case shown="\"Spectra Gryph\"" w221 {
                        tunnel: w220 -> [w226 w230 w233]
                        tunnel: [w225 w229 w232] -> w218
                        frame "Atom Analyzer", Default {
                          (unwired) "C:\\Users\\Raman\\Desktop\\AtomAnalyzer_202011.00_Windows\\AtomAnalyzer\\bin\\AtomAnalyzer.exe"
                          n163 = call <vilib>:"System Exec.vi"("wait until completion? (T)"=TRUE, "error in (no error)"=w226, "command line"="C:\\LPT 2\\LPT\\AtomAnalyzer_202011.00_Windows\\AtomAnalyzer\\bin") -> ("error out"=w225:errorcluster)  [unwired: 5 in, 3 out]
                        }
                        frame "Spectra Gryph" {
                          (unwired) "C:\\Program Files (x86)\\Spectragryph 1.2\\SpectraGryph.exe" ("standard input")
                          n164 = call <vilib>:"System Exec.vi"("wait until completion? (T)"=TRUE, "error in (no error)"=w230, "command line"="C:\\LPT 2\\LPT\\Spectragryph 1.2\\SpectraGryph.exe") -> ("error out"=w229:errorcluster)  [unwired: 5 in, 3 out]
                        }
                        frame "Know It All" {
                          n165 = call <vilib>:"System Exec.vi"("wait until completion? (T)"=TRUE, "error in (no error)"=w233, "command line"="C:\\Program Files\\KnowItAll\\Bin\\KnowItAll.exe") -> ("error out"=w232:errorcluster)  [unwired: 5 in, 3 out]
                        }
                      }
                      n166 = flat-sequence {
                        tunnel: w218 -> [w223]
                        tunnel: [w223] -> w217
                        frame #0 {
                          n167 = local write "INTERACTIVE CONTROLS"(6) -> ()
                        }
                      }
                    }
                    frame "Do Nothing" {
                      n168 = flat-sequence {
                        tunnel: w237 -> [w240]
                        tunnel: [w240] -> w236
                        frame #0 {
                          n169 = Wait (ms)(milliseconds to wait=500) -> ()  [unwired: 1 out]
                        }
                      }
                    }
                  }
                  n170 = local write "Status"("Click an Interactive Control or EXIT INT CNTL to Exit" ("STATUS")) -> ()
                }
              }
            }
            n171 = call "LPT-LQCommSetPower.vi"("LQComm Resource In"=w19, "Set Power (mW)"=0.0, "error in"=w20) -> ("LQComm Resource Out"=w26:refnum<visa-resource-name>, "error out"=w25:errorcluster)  [unwired: 2 out]
            n172 = stacked-sequence {
              frame #0 {
              }
              frame #1 {
              }
            }
            n173 = while {
              tunnel: w26 -> [w73]
              tunnel: w25 -> [w72]
              tunnel: [w69] -> w24
              tunnel: [w68] -> w23
              stop <- w66 stop-if-true
              n174 = call "LPT-LQCommGetPower.vi"("error in"=w72, "LQComm Resource In"=w73) -> ("error out"=w68:errorcluster, "NumericValue"=w67:dbl, "LQComm Resource Out"=w69:refnum<visa-resource-name>)  [unwired: 1 in]
              n175 = Wait (ms)(milliseconds to wait=u32 50) -> ()  [unwired: 1 out]
              n176 = local write "Power Out"(w67) -> ()
              n177 = Less?(x=w67, y=0.5) -> (x < y?=w66:bool)
              n178 = local write "Status"("Powering Down Raman Laser" ("STATUS")) -> ()
            }
            n179 = flat-sequence {
              tunnel: w30 -> [w63]
              tunnel: [w63] -> w20
              tunnel: w28 -> [w62]
              tunnel: [w62] -> w19
              frame #0 {
                n180 = local write "INTERACTIVE CONTROLS"(6) -> ()
              }
            }
            n181 = call "LPT-LQOFF.vi"("error in"=w23, "LQComm Resource In"=w24) -> ("error out"=w22:errorcluster, "LQComm Resource Out"=w27:refnum<visa-resource-name>)  [unwired: 1 in, 1 out]
            n182 = call "LPT-LQCommClose.vi"("error in (no error)"=w22, "LQ Resource In"=w27) -> ("error out"=w31:errorcluster)
            n183 = case shown="True" "ID SPECTRA" {
              tunnel: w31 -> [_ w93]
              frame False {
                n184 = global read "LPT-GUI-MIC-ver 5c GLOBAL 1.0.vi" "SHUTDOWN\nPROGRAM"() -> (w86:bool)
                n185 = stacked-sequence {
                  frame #0 {
                    n186 = local write "Start"(FALSE) -> ()
                  }
                  frame #1 {
                  }
                }
                n187 = local write "EXIT INTERACTIVE\nCONTROL"(FALSE) -> ()
                n188 = local write "ABORT \nLOOP"(FALSE) -> ()
                n189 = case shown="False" w86 {
                  frame False {
                    n190 = local write "Status"("Acquisition Complete - Ready to Acquire") -> ()
                  }
                  frame True {
                  }
                }
              }
              frame True {
                n191 = case shown="\"Spectra Gryph\"" "ANALYSIS PROGRAM" {
                  tunnel: w93 -> [w97 w100 w103]
                  frame "Atom Analyzer", Default {
                    (unwired) "C:\\Users\\Raman\\Desktop\\AtomAnalyzer_202011.00_Windows\\AtomAnalyzer\\bin\\AtomAnalyzer.exe" ("standard input")
                    n192 = call <vilib>:"System Exec.vi"("wait until completion? (T)"=TRUE, "error in (no error)"=w97, "command line"="C:\\LPT 2\\LPT\\AtomAnalyzer_202011.00_Windows\\AtomAnalyzer\\bin\\AtomAnalyzer.exe") -> ()  [unwired: 5 in, 4 out]
                  }
                  frame "Spectra Gryph" {
                    (unwired) "C:\\Program Files (x86)\\Spectragryph 1.2\\SpectraGryph.exe" ("standard input")
                    n193 = call <vilib>:"System Exec.vi"("wait until completion? (T)"=TRUE, "error in (no error)"=w100, "command line"="C:\\LPT 2\\LPT\\Spectragryph 1.2\\SpectraGryph.exe") -> ()  [unwired: 5 in, 4 out]
                  }
                  frame "Know It All" {
                    (unwired) "C:\\Program Files\\KnowItAll\\Bin\\KnowItAll.exe" ("standard input")
                    n194 = call <vilib>:"System Exec.vi"("wait until completion? (T)"=TRUE, "error in (no error)"=w103, "command line"="C:\\LPT 2\\LPT\\KnowItAll\\Bin\\KnowItAll.exe") -> ()  [unwired: 5 in, 4 out]
                  }
                }
                n195 = global read "LPT-GUI-MIC-ver 5c GLOBAL 1.0.vi" "SHUTDOWN\nPROGRAM"() -> (w91:bool)
                n196 = case shown="False" w91 {
                  frame False {
                    n197 = local write "Status"("Acquisition Complete - Ready to Acquire") -> ()
                  }
                  frame True {
                  }
                }
                n198 = local write "Start"(FALSE) -> ()
              }
            }
            "Status" <- "Initializing"
          }
          frame "LIBS" {
            # "Turn off\nfunc. gen"
            # "set power level of LIBS by adjusting the pulse rate until a suitable signal level in the spectrometer is obtained, it is assumed that Raman will be performed first, getting the lens approximately into focus position."
            # "LIBS"
            n199 = flat-sequence {
              tunnel: [w524] -> w376
              tunnel: [w523] -> w375
              tunnel: [w522] -> w374
              tunnel: errorcluster {"status"=FALSE, "code"=0, "source"=""} ("error in") -> [w521]
              tunnel: w376 -> [w566]
              tunnel: w375 -> [w565]
              tunnel: w374 -> [w564]
              tunnel: [errorcluster {"status"=FALSE, "code"=0, "source"=""} ("error constant")] -> w364
              tunnel: [w929] -> w371
              tunnel: w364 -> [w927]
              tunnel: w371 -> [w953]
              tunnel: [w950] -> w377
              frame #0 {
                w537 = FALSE  # Write/Read (Get=true)
                # "Make sure \nfunction gen\nis off"
                # "Starting with\n slow speed"
                n200 = call "labview dds-3x25 LPT.vi"("error in (no error)"=w521, "Frequency"=0) -> ("error out"=w520:errorcluster)  [unwired: 1 in]
                n201 = call "Init.vi"("error in (no error)"=w520, "SPI frequency"=u32 4800000) -> ("error out"=w529:errorcluster, "port out"=w530:u8, "handle"=w531:u16)  [unwired: 6 in, 1 out]
                n202 = call "Spi_Config.vi"("error in (no error)"=w529, "port"=w530, "Handle"=w531) -> ("error out"=w528:errorcluster, "port out"=w526:u8, "handle"=w527:u16)  [unwired: 6 in]
                n203 = call "Set or Get SPI Register_3.vi"("Write data (16 bit)"=u16 16, "Write/Read (Get=true)"=w537, "error in (no error)"=w528, "Register name"=Register_name."Sensor ctrl", "port"=w526, "Handle"=w527) -> ("error out"=w534:errorcluster, "port out"=w533:u8, "handle out"=w532:u16)  [unwired: 2 in, 1 out]
                n204 = local write "Status"("INITIALIZING LIBS") -> ()
                n205 = stacked-sequence {
                  tunnel: w534 -> [w540]
                  tunnel: w533 -> [w542]
                  tunnel: w532 -> [w541]
                  tunnel: [w542] -> w524
                  tunnel: [w541] -> w523
                  tunnel: [w540] -> w522
                  frame #0 {
                    n206 = Wait (ms)(milliseconds to wait=u32 100) -> ()  [unwired: 1 out]
                  }
                }
              }
              frame #1 {
                w567 = Register_name."Serial number"  # Register name
                n207 = while {
                  tunnel: w565 -> [w627]
                  tunnel: w566 -> [w626]
                  tunnel: w564 -> [w625]
                  shift-right: [w624] -> _
                  shift-left: w567 -> [w623]
                  tunnel: [w621] -> w553
                  tunnel: [w620] -> w554
                  tunnel: [w619] -> w555
                  tunnel: [w618] -> w549
                  tunnel: [w617] -> w551
                  tunnel: [w616] -> w550
                  stop <- w618 stop-if-true
                  n208 = case shown="\"Detector type\"" w623 {
                    selector: w623 -> [w630 w638 w647 w673 w684 w699 w710 w718 w737 w748 w759 w770 w781 w792 w803 w814 w825 w836 w847 w863 w874 w885 w896 w907 w919]
                    tunnel: w627 -> [w629 w642 w653 w679 w690 w705 w716 w724 w743 w754 w765 w776 w787 w798 w809 w820 w831 w842 w853 w869 w880 w891 w902 w913 w924]
                    tunnel: w626 -> [w628 w641 w652 w678 w689 w704 w715 w723 w742 w753 w764 w775 w786 w797 w808 w819 w830 w841 w852 w868 w879 w890 w901 w912 w923]
                    tunnel: w625 -> [w632 w640 w651 w677 w688 w703 w714 w722 w741 w752 w763 w774 w785 w796 w807 w818 w829 w840 w851 w867 w878 w889 w900 w911 w922]
                    tunnel: [w630 w639 w650 w674 w685 w700 w711 w730 w738 w749 w760 w771 w782 w793 w804 w815 w826 w837 w848 w864 w875 w886 w897 w908 Register_name."Serial number" ("Register name")] -> w624
                    tunnel: [FALSE FALSE FALSE FALSE FALSE FALSE FALSE FALSE FALSE FALSE FALSE FALSE FALSE FALSE FALSE FALSE FALSE FALSE FALSE FALSE FALSE FALSE FALSE FALSE TRUE] -> w622
                    tunnel: [w632 w637 w649 w675 w686 w701 w712 w731 w739 w750 w761 w772 w783 w794 w805 w816 w827 w838 w849 w865 w876 w887 w898 w909 w920] -> w619
                    tunnel: [w629 w634 w645 w672 w682 w698 w709 w729 w736 w747 w757 w768 w780 w791 w802 w813 w824 w835 w846 w862 w873 w884 w895 w906 w918] -> w621
                    tunnel: [w628 w633 w644 w671 w681 w697 w708 w728 w735 w746 w756 w767 w779 w790 w801 w812 w823 w834 w845 w861 w872 w883 w894 w905 w917] -> w620
                    frame Default {
                    }
                    frame "Serial number" {
                      w639 = Register_name."HW version"  # Register name
                      w643 = TRUE  # Write/Read  (Get=true)
                      n209 = call "Set or Get SPI Register_3.vi"("Write/Read (Get=true)"=w643, "error in (no error)"=w640, "Register name"=w638, "port"=w641, "Handle"=w642) -> ("error out"=w637:errorcluster, "Read Data (16 bit)"=→"*PCB SN":u16, "port out"=w633:u8, "handle out"=w634:u16)  [unwired: 3 in]
                    }
                    frame "HW version" {
                      w650 = Register_name."FW version"  # Register name
                      w654 = TRUE  # Write/Read  (Get=true)
                      n210 = call "Set or Get SPI Register_3.vi"("Write/Read (Get=true)"=w654, "error in (no error)"=w651, "Register name"=w647, "port"=w652, "Handle"=w653) -> ("error out"=w649:errorcluster, "Read Data (16 bit)"=→"*HW version":u16, "port out"=w644:u8, "handle out"=w645:u16)  [unwired: 3 in]
                    }
                    frame "FW version" {
                      w674 = Register_name."Detector type"  # Register name
                      w680 = TRUE  # Write/Read  (Get=true)
                      n211 = call "Set or Get SPI Register_3.vi"("Write/Read (Get=true)"=w680, "error in (no error)"=w677, "Register name"=w673, "port"=w678, "Handle"=w679) -> ("error out"=w675:errorcluster, "Read Data (16 bit)"=w665:u16, "port out"=w671:u8, "handle out"=w672:u16)  [unwired: 3 in]
                      "*FW version" <- w665
                      n212 = Split Number(x=w665) -> (hi(x)=w670:u8, lo(x)=w667:u8)
                      n213 = local write "*FW - Revision"(w667) -> ()
                      n214 = Number To Boolean Array(number=w670) -> (Boolean array=w669:bool[])
                      n215 = Index Array(array=w669) -> (element #1=w664:bool, element #2=w663:bool, element #3=w662:bool, element #4=w661:bool, element #5=w660:bool, element #6=w657:bool, element #7=w656:bool, element #8=w655:bool)  [unwired: 8 in]
                      n216 = Build Array(w664, w663, w662, w661, w660) -> (w668:bool[])
                      n217 = Build Array(w657, w656, w655) -> (w659:bool[])
                      n218 = Boolean Array To Number(Boolean array=w668) -> (number=w666:u32)
                      n219 = Boolean Array To Number(Boolean array=w659) -> (number=w658:u32)
                      n220 = local write "*FW - Variant"(w666) -> ()
                      n221 = local write "*FW - Reserved"(w658) -> ()
                    }
                    frame "Detector type" {
                      w685 = Register_name."Pixel per image"  # Register name
                      w691 = TRUE  # Write/Read  (Get=true)
                      n222 = call "Set or Get SPI Register_3.vi"("Write/Read (Get=true)"=w691, "error in (no error)"=w688, "Register name"=w684, "port"=w689, "Handle"=w690) -> ("error out"=w686:errorcluster, "Read Data (16 bit)"=→"*Detector type":u16, "port out"=w681:u8, "handle out"=w682:u16)  [unwired: 3 in]
                    }
                    frame "Pixel per image" {
                      w700 = Register_name."Calib data chars"  # Register name
                      w706 = TRUE  # Write/Read  (Get=true)
                      n223 = call "Set or Get SPI Register_3.vi"("Write/Read (Get=true)"=w706, "error in (no error)"=w703, "Register name"=w699, "port"=w704, "Handle"=w705) -> ("error out"=w701:errorcluster, "Read Data (16 bit)"=w694:u16, "port out"=w697:u8, "handle out"=w698:u16)  [unwired: 3 in]
                      "*Pixels per image" <- w694
                      n224 = Initialize Array(0.0 ("element"), w694) -> (w693:dbl[])
                      n225 = Initialize Array(1.0 ("element"), w694) -> (w692:dbl[])
                      n226 = local write "Dark spectrum"(w693) -> ()
                      n227 = local write "Ref spectrum"(w692) -> ()
                    }
                    frame "Calib data chars" {
                      w711 = Register_name."Sensor ctrl"  # Register name
                      w717 = TRUE  # Write/Read (Get=true)
                      n228 = call "Set or Get SPI Register_3.vi"("Write/Read (Get=true)"=w717, "error in (no error)"=w714, "Register name"=w710, "port"=w715, "Handle"=w716) -> ("error out"=w712:errorcluster, "Read Data (16 bit)"=→"*Calib data chars":u16, "port out"=w708:u8, "handle out"=w709:u16)  [unwired: 3 in]
                    }
                    frame "Sensor ctrl" {
                      w726 = FALSE  # Write/Read  (Get=true)
                      w730 = Register_name."Sensor exp time LSB"  # Register name
                      w733 = TRUE  # Write/Read  (Get=true)
                      n229 = call "Set or Get SPI Register_3.vi"("Write data (16 bit)"=u16 16, "Write/Read (Get=true)"=w726, "error in (no error)"=w722, "Register name"=w718, "port"=w723, "Handle"=w724) -> ("error out"=w721:errorcluster, "port out"=w720:u8, "handle out"=w719:u16)  [unwired: 2 in, 1 out]
                      n230 = call "Set or Get SPI Register_3.vi"("Write/Read (Get=true)"=w733, "error in (no error)"=w721, "Register name"=w718, "port"=w720, "Handle"=w719) -> ("error out"=w731:errorcluster, "Read Data (16 bit)"=w727:u16, "port out"=w728:u8, "handle out"=w729:u16)  [unwired: 3 in]
                      n231 = local write "*Sensor ctrl"(w727) -> ()
                    }
                    frame "Sensor exp time LSB" {
                      w738 = Register_name."Sensor exp time MSB"  # Register name
                      w744 = TRUE  # Write/Read  (Get=true)
                      n232 = call "Set or Get SPI Register_3.vi"("Write/Read (Get=true)"=w744, "error in (no error)"=w741, "Register name"=w737, "port"=w742, "Handle"=w743) -> ("error out"=w739:errorcluster, "Read Data (16 bit)"=→"Sensor exp time LSB":u16, "port out"=w735:u8, "handle out"=w736:u16)  [unwired: 3 in]
                    }
                    frame "Sensor exp time MSB" {
                      w749 = Register_name."Temperature"  # Register name
                      w755 = TRUE  # Write/Read  (Get=true)
                      n233 = call "Set or Get SPI Register_3.vi"("Write/Read (Get=true)"=w755, "error in (no error)"=w752, "Register name"=w748, "port"=w753, "Handle"=w754) -> ("error out"=w750:errorcluster, "Read Data (16 bit)"=→"Sensor exp time MSB":u16, "port out"=w746:u8, "handle out"=w747:u16)  [unwired: 3 in]
                    }
                    frame "Temperature" {
                      w760 = Register_name."Pixel ready"  # Register name
                      w766 = TRUE  # Write/Read  (Get=true)
                      n234 = call "Set or Get SPI Register_3.vi"("Write/Read (Get=true)"=w766, "error in (no error)"=w763, "Register name"=w759, "port"=w764, "Handle"=w765) -> ("error out"=w761:errorcluster, "Read Data (16 bit)"=→"*Temperature  [counts] \n(12 bit ADC)":u16, "port out"=w756:u8, "handle out"=w757:u16)  [unwired: 3 in]
                    }
                    frame "Pixel ready" {
                      w771 = Register_name."Trigger delay LSB"  # Register name
                      w777 = TRUE  # Write/Read  (Get=true)
                      # "This indicator cannot actually \nbe used in this program"
                      n235 = call "Set or Get SPI Register_3.vi"("Write/Read (Get=true)"=w777, "error in (no error)"=w774, "Register name"=w770, "port"=w775, "Handle"=w776) -> ("error out"=w772:errorcluster, "Read Data (16 bit)"=→"Pixels ready":u16, "port out"=w767:u8, "handle out"=w768:u16)  [unwired: 3 in]
                    }
                    frame "Trigger delay LSB" {
                      w782 = Register_name."Trigger delay MSB"  # Register name
                      w788 = TRUE  # Write/Read  (Get=true)
                      n236 = call "Set or Get SPI Register_3.vi"("Write/Read (Get=true)"=w788, "error in (no error)"=w785, "Register name"=w781, "port"=w786, "Handle"=w787) -> ("error out"=w783:errorcluster, "Read Data (16 bit)"=→"Trigger delay LSB":u16, "port out"=w779:u8, "handle out"=w780:u16)  [unwired: 3 in]
                    }
                    frame "Trigger delay MSB" {
                      w793 = Register_name."ADC PGA"  # Register name
                      w799 = TRUE  # Write/Read  (Get=true)
                      n237 = call "Set or Get SPI Register_3.vi"("Write/Read (Get=true)"=w799, "error in (no error)"=w796, "Register name"=w792, "port"=w797, "Handle"=w798) -> ("error out"=w794:errorcluster, "Read Data (16 bit)"=→"Trigger delay MSB":u16, "port out"=w790:u8, "handle out"=w791:u16)  [unwired: 3 in]
                    }
                    frame "ADC PGA" {
                      w804 = Register_name."ADC offset"  # Register name
                      w810 = TRUE  # Write/Read  (Get=true)
                      n238 = call "Set or Get SPI Register_3.vi"("Write/Read (Get=true)"=w810, "error in (no error)"=w807, "Register name"=w803, "port"=w808, "Handle"=w809) -> ("error out"=w805:errorcluster, "Read Data (16 bit)"=→"*ADC gain [counts]":u16, "port out"=w801:u8, "handle out"=w802:u16)  [unwired: 3 in]
                    }
                    frame "ADC offset" {
                      w815 = Register_name."MPP mode change"  # Register name
                      w821 = TRUE  # Write/Read  (Get=true)
                      n239 = call "Set or Get SPI Register_3.vi"("Write/Read (Get=true)"=w821, "error in (no error)"=w818, "Register name"=w814, "port"=w819, "Handle"=w820) -> ("error out"=w816:errorcluster, "Read Data (16 bit)"=→"*ADC offset [counts]":u16, "port out"=w812:u8, "handle out"=w813:u16)  [unwired: 3 in]
                    }
                    frame "MPP mode change" {
                      w826 = Register_name."DATA READY THRESHOLD"  # Register name
                      w832 = TRUE  # Write/Read  (Get=true)
                      n240 = call "Set or Get SPI Register_3.vi"("Write/Read (Get=true)"=w832, "error in (no error)"=w829, "Register name"=w825, "port"=w830, "Handle"=w831) -> ("error out"=w827:errorcluster, "Read Data (16 bit)"=w822:u16, "port out"=w823:u8, "handle out"=w824:u16)  [unwired: 3 in]
                      n241 = local write "*MPP mode change"(w822) -> ()
                    }
                    frame "DATA READY THRESHOLD" {
                      w837 = Register_name."IMAGES_TO_AVERAGE"  # Register name
                      w843 = TRUE  # Write/Read  (Get=true)
                      n242 = call "Set or Get SPI Register_3.vi"("Write/Read (Get=true)"=w843, "error in (no error)"=w840, "Register name"=w836, "port"=w841, "Handle"=w842) -> ("error out"=w838:errorcluster, "Read Data (16 bit)"=w833:u16, "port out"=w834:u8, "handle out"=w835:u16)  [unwired: 3 in]
                      n243 = local write "*Data ready threshold"(w833) -> ()
                    }
                    frame "IMAGES_TO_AVERAGE" {
                      w848 = Register_name."AVG_CONTROL"  # Register name
                      w854 = TRUE  # Write/Read  (Get=true)
                      n244 = call "Set or Get SPI Register_3.vi"("Write/Read (Get=true)"=w854, "error in (no error)"=w851, "Register name"=w847, "port"=w852, "Handle"=w853) -> ("error out"=w849:errorcluster, "Read Data (16 bit)"=w844:u16, "port out"=w845:u8, "handle out"=w846:u16)  [unwired: 3 in]
                      n245 = local write "*Averaging in HW"(w844) -> ()
                    }
                    frame "AVG_CONTROL" {
                      w864 = Register_name."SPECTROMETER SN"  # Register name
                      w870 = TRUE  # Write/Read  (Get=true)
                      n246 = call "Set or Get SPI Register_3.vi"("Write/Read (Get=true)"=w870, "error in (no error)"=w867, "Register name"=w863, "port"=w868, "Handle"=w869) -> ("error out"=w865:errorcluster, "Read Data (16 bit)"=w860:u16, "port out"=w861:u8, "handle out"=w862:u16)  [unwired: 3 in]
                      n247 = Number To Boolean Array(number=w860) -> (Boolean array=w859:bool[])
                      n248 = Index Array(array=w859, index #1=0 ("index"), index #2=1 ("index")) -> (element #1=w856:bool, element #2=w855:bool)
                      n249 = local write "*Auto trig"(w856) -> ()
                      n250 = local write "Average in progress"(w855) -> ()
                    }
                    frame "SPECTROMETER SN" {
                      w875 = Register_name."SKIPPING_START"  # Register name
                      w881 = TRUE  # Write/Read  (Get=true)
                      n251 = call "Set or Get SPI Register_3.vi"("Write/Read (Get=true)"=w881, "error in (no error)"=w878, "Register name"=w874, "port"=w879, "Handle"=w880) -> ("error out"=w876:errorcluster, "Read Data (16 bit)"=w871:u16, "port out"=w872:u8, "handle out"=w873:u16)  [unwired: 3 in]
                      n252 = local write "*Spectrometer SN"(w871) -> ()
                    }
                    frame "SKIPPING_START" {
                      w886 = Register_name."SKIPPING_END"  # Register name
                      w892 = TRUE  # Write/Read  (Get=true)
                      n253 = call "Set or Get SPI Register_3.vi"("Write/Read (Get=true)"=w892, "error in (no error)"=w889, "Register name"=w885, "port"=w890, "Handle"=w891) -> ("error out"=w887:errorcluster, "Read Data (16 bit)"=w882:u16, "port out"=w883:u8, "handle out"=w884:u16)  [unwired: 3 in]
                      n254 = local write "Skipping start read buffer"(w882) -> ()
                      n255 = local write "*First pixel of interest"(w882) -> ()
                    }
                    frame "SKIPPING_END" {
                      w897 = Register_name."debug"  # Register name
                      w903 = TRUE  # Write/Read  (Get=true)
                      n256 = call "Set or Get SPI Register_3.vi"("Write/Read (Get=true)"=w903, "error in (no error)"=w900, "Register name"=w896, "port"=w901, "Handle"=w902) -> ("error out"=w898:errorcluster, "Read Data (16 bit)"=w893:u16, "port out"=w894:u8, "handle out"=w895:u16)  [unwired: 3 in]
                      n257 = local write "Skipping end read buffer"(w893) -> ()
                      n258 = local write "*Last pixel of interest"(w893) -> ()
                    }
                    frame "debug" {
                      w908 = Register_name."Production mode"  # Register name
                      w914 = TRUE  # Write/Read  (Get=true)
                      n259 = call "Set or Get SPI Register_3.vi"("Write/Read (Get=true)"=w914, "error in (no error)"=w911, "Register name"=w907, "port"=w912, "Handle"=w913) -> ("error out"=w909:errorcluster, "Read Data (16 bit)"=→"Debug":u16, "port out"=w905:u8, "handle out"=w906:u16)  [unwired: 3 in]
                    }
                    frame "Production mode" {
                      w925 = TRUE  # Write/Read  (Get=true)
                      n260 = call "Set or Get SPI Register_3.vi"("Write/Read (Get=true)"=w925, "error in (no error)"=w922, "Register name"=w919, "port"=w923, "Handle"=w924) -> ("error out"=w920:errorcluster, "Read Data (16 bit)"=w916:u16, "port out"=w917:u8, "handle out"=w918:u16)  [unwired: 3 in]
                      n261 = local write "*Production mode"(w916) -> ()
                    }
                  }
                  n262 = local read "Skipping start read buffer"() -> (w617:u16)
                  n263 = local read "Skipping end read buffer"() -> (w616:u16)
                  n264 = Or(x=w619, y=w622) -> (x .or. y?=w618:bool)
                }
                n265 = Equal To 0?(x=w551) -> (x = 0?=w561:bool)
                n266 = Equal To 0?(x=w550) -> (x = 0?=w562:bool)
                n267 = call "Get Calib data.vi"("error in (no error)"=w555, "port"=w554, "Handle"=w553) -> ("error out"=w552:errorcluster, "Cal coef"=w556:dbl[], "port out"=w546:u8, "handle out"=w547:u16)  [unwired: 4 in]
                n268 = stacked-sequence {
                  tunnel: w552 -> [_ _ _ w590 _ _]
                  tunnel: [_ _ _ w590 _ _] -> _
                  tunnel: [_ _ _ w589 _ _] -> w545
                  frame #0 {
                    # "Only CCD supports MPP"
                    n269 = local read "*Detector type"() -> (w568:u16)
                    n270 = case shown="0, Default" w568 {
                      frame 0, Default {
                        # "CMOS-type"
                        n271 = property on="*MPP mode change" class="DigNum (strict)"("DisabledEnum"=T9."Disabled and Grayed Out" ("Disabled")) -> ()  [unwired: 2 in, 2 out]
                      }
                      frame 1 {
                        # "CCD type S11156"
                        n272 = property on="*MPP mode change" class="DigNum (strict)"("DisabledEnum"=T9."Enabled" ("Disabled")) -> ()  [unwired: 2 in, 2 out]
                      }
                    }
                  }
                  frame #1 {
                    # "Time per clock: Slow CMOS?"
                    n273 = local read "*Detector type"() -> (w576:u16)
                    n274 = local read "*FW - Variant"() -> (w575:u16)
                    n275 = Equal To 0?(x=w576) -> (x = 0?=w572:bool)
                    n276 = Equal?(x=w575, y=u16 2) -> (x = y?=w573:bool)
                    n277 = And(x=w572, y=w573) -> (x .and. y?=w571:bool)
                    n278 = case shown="False" w571 {
                      frame False {
                        # "Full speed for everything else\nUnless slowed down again..."
                        n279 = local write "SPI clock frequency [Hz]"(u32 24000000 ("SPI clock frequency [Hz]")) -> ()
                      }
                      frame True {
                        n280 = local write "msPerClock"(0.001 ("msPerClock")) -> ()
                        n281 = local write "SPI clock frequency [Hz]"(u32 4800000 ("SPI clock frequency [Hz]")) -> ()
                      }
                    }
                  }
                  frame #2 {
                    # "Time per clock: Slow CCD?"
                    n282 = local read "*Detector type"() -> (w581:u16)
                    n283 = local read "*FW - Variant"() -> (w586:u16)
                    n284 = Equal?(x=u16 1 ("y"), y=w581) -> (x = y?=w580:bool)
                    n285 = Equal?(x=w586, y=u16 1) -> (x = y?=w583:bool)
                    n286 = And(x=w580, y=w583) -> (x .and. y?=w584:bool)
                    n287 = case shown="True" w584 {
                      frame False {
                      }
                      frame True {
                        n288 = local write "msPerClock"(0.0004 ("msPerClock")) -> ()
                        n289 = local write "SPI clock frequency [Hz]"(u32 12000000 ("SPI clock frequency [Hz]")) -> ()
                      }
                    }
                  }
                  frame #3 {
                    # "Set SPI speed"
                    n290 = local read "SPI clock frequency [Hz]"() -> (w589:u32)
                  }
                  frame #4 {
                    # "Premium features: DISB-101S"
                    n291 = local read "*Detector type"() -> (w596:u16)
                    n292 = local read "*FW - Variant"() -> (w595:u16)
                    n293 = Equal To 0?(x=w596) -> (x = 0?=w592:bool)
                    n294 = Equal?(x=w595, y=u16 1) -> (x = y?=w593:bool)
                    n295 = And(x=w592, y=w593) -> (x .and. y?=w591:bool)
                    n296 = case shown="True" w591 {
                      frame False {
                      }
                      frame True {
                        n297 = property on="*First pixel of interest" class="DigNum (strict)"("DisabledEnum"=T9."Enabled" ("Disabled")) -> ()  [unwired: 2 in, 2 out]
                        n298 = property on="*Last pixel of interest" class="DigNum (strict)"("DisabledEnum"=T9."Enabled" ("Disabled")) -> ()  [unwired: 2 in, 2 out]
                      }
                    }
                  }
                  frame #5 {
                  }
                }
                n299 = And(x=w561, y=w562) -> (x .and. y?=w563:bool)
                n300 = stacked-sequence {
                  tunnel: w556 -> [w612]
                  tunnel: [w610] -> w559
                  tunnel: [w609] -> w557
                  tunnel: w549 -> [_]
                  frame #0 {
                    n301 = local read "*Pixels per image"() -> (w611:u16)
                    n302 = for {
                      N: w611 -> [_]
                      tunnel: w612 -> [w615]
                      tunnel: [w614] -> w609 mode=indexing
                      tunnel: [w613] -> w610 mode=indexing
                      i -> [w613]
                      n303 = call "Pix_lamda_Poly_conversion.vi"("Pixels"=w613, "Cal coef"=w615) -> ("Lamda(nm)"=w614:dbl)  [unwired: 7 in, 6 out]
                    }
                  }
                }
                n304 = local write "*Cal coef"(w556) -> ()
                n305 = case shown="True" w563 {
                  tunnel: w557 -> [w606 w607]
                  tunnel: [w604 w607] -> w558
                  tunnel: w559 -> [w602 w608]
                  tunnel: [w601 w608] -> w560
                  tunnel: w550 -> [w600 _]
                  tunnel: w551 -> [w599 _]
                  frame False {
                    n306 = Subtract(x=w600, y=w599) -> (x-y=w605:u16)
                    n307 = Increment(x=w605) -> (x+1=w603:u16)
                    n308 = Array Subset(array=w606, index=w599, length=w603) -> (w604:dbl[])
                    n309 = Array Subset(array=w602, index=w599, length=w603) -> (w601:i32[])
                  }
                  frame True {
                  }
                }
                n310 = local write "*Wavelength axis"(w558) -> ()
                n311 = call "Spi_Set Frequency.vi"("error in (no error)"=errorcluster {"status"=FALSE, "code"=0, "source"=""} ("error constant"), "Frequency"=w545, "port"=w546, "Handle"=w547) -> ("Actual frequency"=w548:u32)  [unwired: 4 in, 3 out]
                n312 = local write "SPI clock frequency [Hz]"(w548) -> ()
                n313 = local write "Pixel axis"(w560) -> ()
              }
              frame #2 {
                # "take dark scan, save to file, or zero dark scan"
                n314 = local read "Get Dark?"() -> (w928:bool)
                n315 = case shown="False" w928 {
                  tunnel: [w939 w946] -> w929
                  tunnel: [w931 "Zero Dark LIBS"] -> w926
                  tunnel: w927 -> [w932 w947]
                  frame True {
                    n316 = Format Date/Time String(time format string (%c)="%y%m%d%H%M%S") -> (date/time string=w936:string)  [unwired: 2 in]
                    n317 = Concatenate Strings(w936, "LIBS" ("string"), "Dark" ("string")) -> (w938:string)
                    n318 = Build Path(base path=path "C:/Program Files (x86)/National Instruments/LabVIEW 2019/instr.lib/LPT/DataLIBS", name or relative path=w938) -> (appended path=w942:path)
                    n319 = call "LPT-LIBS-Spectra Acquire.vi"("error in"=w932) -> ("error out"=w940:errorcluster, "Raw Data"=w931:dbl[])  [unwired: 7 in, 2 out]
                    n320 = call-poly <vilib>:"Write Delimited Spreadsheet.vi"("file path (dialog if empty)"=w942, "1D data"=w931, "error in (no error)"=w940, "transpose? (no:F)"=TRUE) -> ("error out"=w939:errorcluster)  [unwired: 10 in, 1 out]
                  }
                  frame False {
                    n321 = local read "Start"() -> (w945:bool)
                    n322 = call "LPT-FileSave.vi"("error in (no error)"=w947, "Data\\Dark"=FALSE ("Data\\Dark"), "Raman\\LIBS"=w945, "Array"="Zero Dark LIBS") -> ("error out"=w946:errorcluster)  [unwired: 7 in]
                  }
                }
                "LIBS Dark Spectra" <- w926
                n323 = case shown="False" w928 {
                  frame False {
                  }
                  frame True {
                    n324 = local write "Status"("Getting Dark Spectrum") -> ()
                  }
                }
              }
              frame #3 {
                # "set power, verify power, auto focus"
                n325 = case shown="False" "Auto Set\nLaser Frequency" {
                  tunnel: w953 -> [w1044 w1046]
                  tunnel: [w1043 w1045] -> w951
                  frame False {
                    n326 = call "labview dds-3x25 LPT.vi"("error in (no error)"=w1044, "Frequency"="LIBS Laser Frequency (Hz)") -> ("error out"=w1043:errorcluster)  [unwired: 1 in]
                    n327 = Number To Decimal String(number="LIBS Laser Frequency (Hz)") -> (decimal integer string=w1040:string)  [unwired: 1 in]
                    n328 = Concatenate Strings("Setting LIBS Laser Frequency to ", w1040) -> (w1042:string)
                    n329 = local write "Status"(w1042) -> ()
                  }
                  frame True {
                    n330 = while {
                      tunnel: w1046 -> [w1049]
                      tunnel: [w1059] -> w1045
                      i -> [w1053]
                      stop <- w1050 stop-if-true
                      n331 = local read "LIBS Dark Spectra"() -> (w1061:dbl[])
                      n332 = Multiply(x=w1053, y=90) -> (x*y=w1047:i32)
                      n333 = call "labview dds-3x25 LPT.vi"("error in (no error)"=w1049, "Frequency"=w1047) -> ("error out"=w1048:errorcluster)  [unwired: 1 in]
                      n334 = Equal?(x=w1053, y=10) -> (x = y?=w1051:bool)
                      n335 = call "LPT-LIBS-Spectra Acquire.vi"("error in"=w1048, "LIBS Dark Array"=w1061) -> ("error out"=w1059:errorcluster, "Raw Data"=w1060:dbl[])  [unwired: 6 in, 2 out]
                      n336 = case shown="True" w1051 {
                        frame False {
                        }
                        frame True {
                          n337 = One Button Dialog(message="No/Poor signal") -> ()  [unwired: 1 in, 1 out]
                        }
                      }
                      n338 = Array Max & Min(array=w1060) -> (max value=w1055:dbl)  [unwired: 3 out]
                      n339 = local write "Status"("Auto Setting Laser Frequency") -> ()
                      n340 = Greater?(x=w1055, y=3000.0) -> (0:w1056:bool)
                      n341 = Or(x=w1056, y=w1051) -> (x .or. y?=w1050:bool)
                    }
                  }
                }
                n342 = local read "AUT FOCUS"() -> (w952:bool)
                n343 = case shown="False" FALSE {
                  tunnel: w952 -> [w954 w1009]
                  tunnel: w951 -> [w956 w1008]
                  tunnel: [w955 w1007] -> w950
                  frame False {
                    n344 = case shown="True" w954 {
                      tunnel: w956 -> [w957 w959]
                      tunnel: [w957 w958] -> w955
                      frame False {
                      }
                      frame True {
                        n345 = stacked-sequence {
                          seq-local: [w962 _ _] -> [_ w996 _]
                          seq-local: [w961 _ _] -> [_ w999 _]
                          seq-local: ["STAGE START 2" _ _] -> [_ w1000 _]
                          tunnel: [w964 _ _] -> w958
                          tunnel: w959 -> [w964 _ _]
                          frame #0 {
                            n346 = Subtract(x="STAGE STOP 2", y="STAGE START 2") -> (x-y=w966:i32)
                            n347 = Divide(x=w966, y="#of steps 3") -> (x/y=w961:dbl)
                            n348 = Increment(x="#of steps 3") -> (x+1=w967:i32)
                            n349 = for {
                              N: w967 -> [_]
                              tunnel: w961 -> [w977]
                              tunnel: "STAGE START 2" -> [w973]
                              shift-right: [w969] -> w962
                              shift-left: sgl[] [] -> [w970]
                              i -> [w976]
                              n350 = stacked-sequence {
                                tunnel: [_ w979] -> w971
                                frame #0 {
                                n351 = Wait (ms)(milliseconds to wait=u32 1000) -> ()  [unwired: 1 out]
                                }
                                frame #1 {
                                n352 = call "LPT-SpectraWiz-Acquire W Dark.vi"() -> ("Buffer"=w979:sgl[])  [unwired: 10 in, 1 out]
                                }
                              }
                              "Raw Data 2" <- w971
                              n353 = Multiply(x=w977, y=w976) -> (x*y=w975:dbl)
                              n354 = Add(x=w973, y=w975) -> (x+y=w974:dbl)
                              n355 = stacked-sequence {
                                tunnel: w974 -> [_ w983 _ _ _]
                                frame #0 {
                                n356 = local write "AUT FOCUS STATUS 2"(FALSE ("AUT FOCUS STATUS 2")) -> ()
                                }
                                frame #1 {
                                n357 = Number To Decimal String(number=w983) -> (decimal integer string=w982:string)  [unwired: 1 in]
                                "NUMBER 2" <- w982
                                n358 = Concatenate Strings("DPOS=", w982) -> (→"COMMAND 3":string)
                                "Position (um) 2" <- w983
                                }
                                frame #2 {
                                n359 = local read "COMMAND 3"() -> (w988:string)
                                n360 = call "Serial Write and Read on Two Ports 3.0.vi"("Write String"=w988) -> ("Read String"=w985:string)  [unwired: 10 in]
                                "COMMAND1 READ 3" <- w985
                                n361 = local read "NUMBER 2"() -> (w987:string)
                                n362 = Match Pattern(string=w985, regular expression=w987) -> ()  [unwired: 1 in, 4 out]
                                n363 = Equal?(x=w985, y=w985) -> (x = y?=→"AUT FOCUS STATUS 2":bool)
                                }
                                frame #3 {
                                n364 = local read "COMMAND1 READ 3"() -> (w989:string)
                                n365 = Match Pattern(string=w989, regular expression="EPOS=") -> (after substring=w993:string)  [unwired: 1 in, 3 out]
                                n366 = Match Pattern(string=w993, regular expression="\\n") -> (before substring=w991:string)  [unwired: 1 in, 3 out]
                                n367 = Decimal String To Number(string=w991) -> (number=w990:i32)  [unwired: 2 in, 1 out]
                                n368 = local write "Position (um)"(w990) -> ()
                                }
                                frame #4 {
                                n369 = Wait (ms)(milliseconds to wait=u32 100) -> ()  [unwired: 1 out]
                                }
                              }
                              n370 = Add Array Elements(numeric array=w971) -> (sum=w972:sgl)
                              "power sum 2" <- w972
                              n371 = Build Array (concatenate)(w970, w972) -> (w969:sgl[])
                            }
                          }
                          frame #1 {
                            (unwired) 10.0 ("Position (mm)")
                            (unwired) 500.0 ("MaxPosition")
                            (unwired) sgl 3651732.0 ("max value")
                            n372 = Array Max & Min(array=w996) -> (max value=w998:sgl, max index (indices)=w1002:i32)  [unwired: 2 out]
                            n373 = Multiply(x=w1002, y=w999) -> (x*y=w1001:dbl)
                            n374 = local write "max value"(w998) -> ()
                            n375 = Add(x=w1001, y=w1000) -> (x+y=w997:dbl)
                            n376 = local write "Position (um) 2"(w997) -> ()
                            n377 = local write "MaxPosition"(w997) -> ()
                          }
                          frame #2 {
                            n378 = local read "Position (um) 2"() -> (w1004:dbl)
                            n379 = Number To Decimal String(number=w1004) -> (decimal integer string=w1005:string)  [unwired: 1 in]
                            n380 = Concatenate Strings("MOV ", w1005) -> (w1003:string)
                            n381 = call "Serial Write and Read on Two Ports 3.0.vi"("Write String"=w1003) -> ()  [unwired: 10 in, 1 out]
                          }
                        }
                      }
                    }
                  }
                  frame True {
                    n382 = case shown="True" w1009 {
                      tunnel: w1008 -> [w1010 w1020]
                      tunnel: [w1010 w1011] -> w1007
                      frame False {
                      }
                      frame True {
                        n383 = local read "LED 1 STATUS"() -> (w1013:bool)
                        n384 = local read "Set End Position (um)"() -> (w1017:dbl)
                        n385 = case shown="True" w1013 {
                          tunnel: w1017 -> [_ w1033]
                          tunnel: [w1025 w1030] -> w1016
                          tunnel: [w1024 10] -> w1015
                          tunnel: [w1023 w1029] -> w1014
                          frame False {
                            n386 = local read "#of steps A"() -> (w1024:i32)
                            n387 = local read "STAGE STOP A"() -> (w1023:i32)
                            n388 = local read "STAGE START A"() -> (w1025:i32)
                          }
                          frame True {
                            n389 = Subtract(x=w1033, y=1) -> (x-y=w1026:dbl)
                            n390 = Less?(x=w1026, y=1) -> (x < y?=w1028:bool)
                            n391 = case shown="False" w1028 {
                              tunnel: w1026 -> [w1035 _]
                              tunnel: [w1035 1] -> w1030
                              tunnel: [w1034 3] -> w1029
                              frame False {
                                n392 = Add(x=2, y=w1035) -> (x+y=w1034:dbl)
                              }
                              frame True {
                              }
                            }
                          }
                        }
                        n393 = local read "LIBS Dark Spectra"() -> (w1018:dbl[])
                        n394 = call "LPT-Actuonix-LIBS-AutoFocus.vi"("LIBS Dark Array"=w1018, "error in (no error)"=w1020, "STOP"=w1014, "START"=w1016, "#of steps"=w1015) -> ("error out"=w1012:errorcluster, "Position (mm)"=w1019:dbl)  [unwired: 2 in, 3 out]
                        n395 = local write "Set End Position (um)"(w1019) -> ()
                        n396 = in-place {
                          in-place-border: w1012 -> [w1022]
                          in-place-border: [w1022] -> w1011
                          n397 = local write "LED 1 STATUS"(TRUE) -> ()
                        }
                      }
                    }
                  }
                }
                n398 = case shown="False" w952 {
                  frame False {
                  }
                  frame True {
                    n399 = local write "Status"("Autofocus") -> ()
                  }
                }
              }
            }
            n400 = local read "AutoAcquire"() -> (w372:bool)
            n401 = case shown="True" w372 {
              tunnel: [w400 w412] -> w366
              tunnel: w377 -> [w397 w411]
              frame True {
                n402 = local read "Number of Scans  to Acquire"() -> (w398:i32)
                n403 = call "LPT-ImageSnapandSave.vi"("error in"=w397, "Raman\\LIBS"=FALSE ("Raman\\LIBS")) -> ("error out"=w396:errorcluster)  [unwired: 9 in]
                n404 = for {
                  N: w398 -> [_]
                  shift-right: [w405] -> w400
                  shift-left: w396 -> [w403]
                  w407 = FALSE ("Raman\\LIBS")
                  n405 = local read "LIBS Dark Spectra"() -> (w401:dbl[])
                  n406 = call "LPT-LIBS-Spectra Acquire.vi"("error in"=w403, "LIBS Dark Array"=w401) -> ("error out"=w409:errorcluster, "Removed background"=→"Removed background":dbl[], "Raw Data"=w410:dbl[], "Spectrum"=w404:cluster{dbl[], dbl[]})  [unwired: 6 in]
                  n407 = local write "Spectrum"(w404) -> ()
                  n408 = call "LPT-FileSave.vi"("error in (no error)"=w409, "Data\\Dark"=TRUE ("Data\\Dark"), "Raman\\LIBS"=w407, "Array"=w410) -> ("error out"=w406:errorcluster)  [unwired: 7 in]
                  n409 = call "LPT-XYFileSave.vi"("error in (no error)"=w406, "Raman\\LIBS"=w407, "Spectrum"=w404) -> ("error out"=w405:errorcluster)  [unwired: 8 in]
                }
                n410 = local write "Status"("Aquiring Spectrum" ("STATUS")) -> ()
              }
              frame False {
                n411 = while {
                  tunnel: [w416] -> w412
                  tunnel: w411 -> [w417]
                  stop <- w414 stop-if-true
                  n412 = local read "INTERACTIVE CONTROLS"() -> (w418:T3)
                  n413 = case shown="\"ReFocus\"" w418 {
                    tunnel: w417 -> [w427 w438 w459 w482 w493 w499 w516]
                    tunnel: [w428 w436 w457 w480 w492 w497 w515] -> w416
                    frame "Acquire" {
                      n414 = call "LPT-ImageSnapandSave.vi"("error in"=w427, "Raman\\LIBS"=FALSE) -> ("error out"=w425:errorcluster)  [unwired: 9 in]
                      n415 = local read "LIBS Dark Spectra"() -> (w433:dbl[])
                      n416 = call "LPT-LIBS-Spectra Acquire.vi"("error in"=w425, "LIBS Dark Array"=w433) -> ("error out"=w431:errorcluster, "Removed background"=w424:dbl[], "Raw Data"=w432:dbl[], "Spectrum"=w421:cluster{dbl[], dbl[]})  [unwired: 6 in]
                      n417 = local write "Removed background"(w424) -> ()
                      n418 = local write "Spectrum"(w421) -> ()
                      n419 = call "LPT-FileSave.vi"("error in (no error)"=w431, "Data\\Dark"=TRUE ("Data\\Dark"), "Raman\\LIBS"=FALSE ("Raman\\LIBS"), "Array"=w432) -> ("error out"=w423:errorcluster)  [unwired: 7 in]
                      n420 = call "LPT-XYFileSave.vi"("error in (no error)"=w423, "Raman\\LIBS"=FALSE, "Spectrum"=w421) -> ("error out"=w422:errorcluster)  [unwired: 8 in]
                      n421 = flat-sequence {
                        tunnel: w422 -> [w434]
                        tunnel: [w434] -> w428
                        frame #0 {
                          n422 = Wait (ms)(milliseconds to wait=1000) -> ()  [unwired: 1 out]
                        }
                      }
                    }
                    frame "ReFocus" {
                      n423 = local read "Set End Position (um)"() -> (w446:dbl)
                      n424 = Subtract(x=w446, y=1) -> (x-y=w442:dbl)
                      n425 = Less?(x=w442, y=1) -> (x < y?=w443:bool)
                      n426 = case shown="False" w443 {
                        tunnel: [w454 1] -> w444
                        tunnel: [w453 3] -> w445
                        tunnel: w442 -> [w454 _]
                        frame False {
                          n427 = Add(x=2, y=w454) -> (x+y=w453:dbl)
                        }
                        frame True {
                        }
                      }
                      n428 = local read "LIBS Dark Spectra"() -> (w447:dbl[])
                      n429 = call "LPT-Actuonix-LIBS-AutoFocus.vi"("LIBS Dark Array"=w447, "error in (no error)"=w438, "STOP"=w445, "START"=w444, "#of steps"=10) -> ("error out"=w437:errorcluster, "Position (mm)"=w448:dbl)  [unwired: 2 in, 3 out]
                      n430 = local write "Set End Position (um)"(w448) -> ()
                      n431 = flat-sequence {
                        tunnel: w437 -> [w450]
                        tunnel: [w450] -> _
                        tunnel: [w450] -> w436
                        frame #0 {
                          n432 = local write "INTERACTIVE CONTROLS"(6) -> ()
                          n433 = Wait (ms)(milliseconds to wait=1000) -> ()  [unwired: 1 out]
                        }
                      }
                    }
                    frame "ReSet Power" {
                      n434 = while {
                        tunnel: [w475] -> w458
                        tunnel: w459 -> [w469]
                        i -> [w466]
                        stop <- w470 stop-if-true
                        n435 = local read "power setting from LQ"() -> (w474:string)
                        n436 = Multiply(x=w466, y=100) -> (x*y=w464:i32)
                        n437 = local read "LIBS Dark Spectra"() -> (w478:dbl[])
                        n438 = Equal?(x=w466, y=10) -> (x = y?=w463:bool)
                        n439 = call "LPT-LIBS-Burst Mod.vi"("Delay (50ms)"=50, "Frequency (10 Hz)"=w464, "error in (no error)"=w469, "VISA resource name"=w474) -> ("error out"=w477:errorcluster)  [unwired: 6 in, 1 out]
                        n440 = case shown="True" w463 {
                          frame False {
                          }
                          frame True {
                            n441 = One Button Dialog(message="No/Poor signal") -> ()  [unwired: 1 in, 1 out]
                          }
                        }
                        n442 = call "LPT-LIBS-Spectra Acquire.vi"("error in"=w477, "LIBS Dark Array"=w478) -> ("error out"=w475:errorcluster, "Raw Data"=w476:dbl[])  [unwired: 6 in, 2 out]
                        n443 = Array Max & Min(array=w476) -> (max value=w471:dbl)  [unwired: 3 out]
                        n444 = Greater?(x=w471, y=3000.0) -> (0:w473:bool)
                        n445 = Or(x=w473, y=w463) -> (x .or. y?=w470:bool)
                      }
                      n446 = flat-sequence {
                        tunnel: [w460] -> w457
                        tunnel: w458 -> [w460]
                        frame #0 {
                          n447 = local write "INTERACTIVE CONTROLS"(6) -> ()
                          n448 = Wait (ms)(milliseconds to wait=1000) -> ()  [unwired: 1 out]
                        }
                      }
                    }
                    frame "New Dark" {
                      n449 = stacked-sequence {
                        tunnel: w482 -> [w489]
                        tunnel: [w490] -> w481
                        frame #0 {
                          n450 = call "LPT-SpectraWiz-GetDark.vi"("error in"=w489) -> ("error out"=w491:errorcluster, "Dark Spectra"=w486:sgl[])  [unwired: 9 in]
                          n451 = local write "LIBS Dark Spectra"(w486) -> ()
                          n452 = call "LPT-FileSave.vi"("error in (no error)"=w491, "Data\\Dark"=FALSE ("Data\\Dark"), "Raman\\LIBS"=FALSE ("Raman\\LIBS"), "Array"=w486) -> ("error out"=w490:errorcluster)  [unwired: 7 in]
                        }
                      }
                      n453 = flat-sequence {
                        tunnel: w481 -> [w484]
                        tunnel: [w484] -> w480
                        frame #0 {
                          n454 = local write "INTERACTIVE CONTROLS"(6) -> ()
                          n455 = Wait (ms)(milliseconds to wait=1000) -> ()  [unwired: 1 out]
                        }
                      }
                    }
                    frame "Parameter Reset" {
                      n456 = flat-sequence {
                        tunnel: w493 -> [w494]
                        tunnel: [w494] -> w492
                        frame #0 {
                          n457 = local write "INTERACTIVE CONTROLS"(6) -> ()
                          n458 = Wait (ms)(milliseconds to wait=500) -> ()  [unwired: 1 out]
                        }
                      }
                    }
                    frame "Material ID" {
                      n459 = local read "ANALYSIS PROGRAM"() -> (w500:T4)
                      n460 = case shown="\"Atom Analyzer\", Default" w500 {
                        tunnel: w499 -> [w505 w508 w513]
                        tunnel: [w504 w507 w512] -> w498
                        frame "Atom Analyzer", Default {
                          (unwired) "C:\\Users\\Raman\\Desktop\\AtomAnalyzer_202011.00_Windows\\AtomAnalyzer\\bin\\AtomAnalyzer.exe"
                          n461 = call <vilib>:"System Exec.vi"("wait until completion? (T)"=TRUE, "error in (no error)"=w505, "command line"="C:\\LPT 2\\LPT\\AtomAnalyzer_202011.00_Windows\\AtomAnalyzer\\bin\\AtomAnalyzer.exe") -> ("error out"=w504:errorcluster)  [unwired: 5 in, 3 out]
                        }
                        frame "Spectra Gryph" {
                          n462 = call <vilib>:"System Exec.vi"("wait until completion? (T)"=TRUE, "error in (no error)"=w508, "command line"="C:\\Program Files (x86)\\Spectragryph 1.2\\SpectraGryph.exe" ("standard input")) -> ("error out"=w507:errorcluster)  [unwired: 5 in, 3 out]
                        }
                        frame "Know It All" {
                          (unwired) "C:\\Program Files\\KnowItAll\\Bin\\KnowItAll.exe"
                          n463 = call <vilib>:"System Exec.vi"("wait until completion? (T)"=TRUE, "error in (no error)"=w513, "command line"="C:\\LPT 2\\LPT\\KnowItAll\\Bin\\KnowItAll.exe") -> ("error out"=w512:errorcluster)  [unwired: 5 in, 3 out]
                        }
                      }
                      n464 = flat-sequence {
                        tunnel: w498 -> [w501]
                        tunnel: [w501] -> w497
                        frame #0 {
                          n465 = local write "INTERACTIVE CONTROLS"(6) -> ()
                        }
                      }
                    }
                    frame "Do Nothing", Default {
                      n466 = flat-sequence {
                        tunnel: w516 -> [w517]
                        tunnel: [w517] -> _
                        tunnel: [w517] -> w515
                        frame #0 {
                          n467 = Wait (ms)(milliseconds to wait=500) -> ()  [unwired: 1 out]
                        }
                      }
                    }
                  }
                  n468 = local write "Status"("Click an Interactive Control or EXIT INT CNTL to Exit" ("STATUS")) -> ()
                  n469 = local read "EXIT INTERACTIVE\nCONTROL"() -> (w415:bool)
                  n470 = local read "SHUTDOWN\nPROGRAM"() -> (w413:bool)
                  n471 = Or(x=w415, y=w413) -> (x .or. y?=w414:bool)
                }
              }
            }
            n472 = flat-sequence {
              tunnel: w366 -> [w378]
              tunnel: [w378] -> w365
              frame #0 {
                n473 = local write "INTERACTIVE CONTROLS"(6) -> ()
              }
            }
            n474 = local read "ID SPECTRA"() -> (w373:bool)
            n475 = case shown="True" w373 {
              tunnel: w368 -> [_ w384]
              frame False {
              }
              frame True {
                n476 = local read "ANALYSIS PROGRAM"() -> (w385:T4)
                n477 = case shown="\"Atom Analyzer\", Default" w385 {
                  tunnel: w384 -> [w387 w391 w394]
                  frame "Atom Analyzer", Default {
                    (unwired) "C:\\Users\\Raman\\Desktop\\AtomAnalyzer_202011.00_Windows\\AtomAnalyzer\\bin\\AtomAnalyzer.exe" ("standard input")
                    n478 = call <vilib>:"System Exec.vi"("wait until completion? (T)"=TRUE, "error in (no error)"=w387, "command line"="C:\\LPT 2\\LPT\\AtomAnalyzer_202011.00_Windows\\AtomAnalyzer\\bin\\AtomAnalyzer.exe") -> ()  [unwired: 5 in, 4 out]
                  }
                  frame "Spectra Gryph" {
                    n479 = call <vilib>:"System Exec.vi"("wait until completion? (T)"=TRUE, "error in (no error)"=w391, "command line"="C:\\Program Files (x86)\\Spectragryph 1.2\\SpectraGryph.exe" ("standard input")) -> ()  [unwired: 5 in, 4 out]
                  }
                  frame "Know It All" {
                    n480 = call <vilib>:"System Exec.vi"("wait until completion? (T)"=TRUE, "error in (no error)"=w394, "command line"="C:\\Program Files\\KnowItAll\\Bin\\KnowItAll.exe" ("standard input")) -> ()  [unwired: 5 in, 4 out]
                  }
                }
              }
            }
            n481 = call "labview dds-3x25 LPT.vi"("error in (no error)"=w365, "Frequency"=0) -> ("error out"=w369:errorcluster)  [unwired: 1 in]
            n482 = flat-sequence {
              tunnel: w369 -> [w381]
              tunnel: [w381] -> w368
              frame #0 {
                n483 = local write "EXIT INTERACTIVE\nCONTROL"(FALSE) -> ()
                n484 = local write "Start"(FALSE) -> ()
                n485 = local write "Status"("Acquisition Complete - Ready to Acquire") -> ()
              }
            }
          }
        }
      }
    }
    n486 = local read "SHUTDOWN\nPROGRAM"() -> (w13:bool)
    "Numeric 7" <- w12
  }
  n487 = case shown="True" TRUE {
    frame False {
    }
    frame True {
      n488 = while {
        i -> [w1064]
        stop <- w1065 stop-if-true
        n489 = stacked-sequence {
          frame #0 {
            n490 = Wait (ms)(milliseconds to wait=u32 10) -> ()  [unwired: 1 out]
          }
          frame #1 {
            w1067 = FALSE ("LED 2")
            n491 = feedback #1(w1067) -> (w1075:bool)
            n492 = Equal?(x="LED 1", y=w1075) -> (x = y?=w1072:bool)
            n493 = feedback-in #1("LED 1") -> ()
            n494 = feedback #2(w1067) -> (w1074:bool)
            n495 = Equal?(x="LED 2", y=w1074) -> (x = y?=w1071:bool)
            n496 = feedback-in #2("LED 2") -> ()
            n497 = case shown="True" w1071 {
              tunnel: "LED 2" -> [w1082 _]
              frame False {
                n498 = case shown="True" w1082 {
                  tunnel: ["LED2 OFF" "LED2 ON"] -> w1081
                  frame False {
                  }
                  frame True {
                  }
                }
                n499 = local write "COMMAND 1"(w1081) -> ()
              }
              frame True {
              }
            }
            n500 = case shown="True" w1072 {
              tunnel: "LED 1" -> [w1086 _]
              frame False {
                n501 = case shown="True" w1086 {
                  tunnel: ["LED1 OFF" "LED1 ON"] -> w1085
                  frame False {
                  }
                  frame True {
                  }
                }
                n502 = local write "COMMAND 1"(w1085) -> ()
              }
              frame True {
              }
            }
            n503 = Not(x=w1072) -> (.not. x?=w1069:bool)
            n504 = Not(x=w1071) -> (.not. x?=w1070:bool)
            n505 = Compound Arithmetic op=OR(w1069, w1070) -> (w1068:bool)
            n506 = stacked-sequence {
              tunnel: w1068 -> [w1077]
              frame #0 {
                n507 = case shown="False" w1077 {
                  frame False {
                  }
                  frame True {
                    n508 = call "Serial Write and Read on Two Ports 3.0.vi"("VISA Resource (write)"="LED", "Write String"="COMMAND 1") -> ("Read String"=→"COMMAND1 READ":string)  [unwired: 9 in]
                  }
                }
              }
            }
          }
          frame #2 {
            w1093 = "LED2 OFF" ("y")
            w1092 = "LED2 ON" ("y")
            w1091 = "LED1 OFF" ("y")
            w1090 = "LED1 ON" ("y")
            n509 = local read "COMMAND1 READ"() -> (w1089:string)
            n510 = Match Pattern(string=w1089, regular expression=w1093) -> (match substring=w1098:string)  [unwired: 1 in, 3 out]
            n511 = Match Pattern(string=w1089, regular expression=w1092) -> (match substring=w1099:string)  [unwired: 1 in, 3 out]
            n512 = Match Pattern(string=w1089, regular expression=w1091) -> (match substring=w1100:string)  [unwired: 1 in, 3 out]
            n513 = Match Pattern(string=w1089, regular expression=w1090) -> (match substring=w1101:string)  [unwired: 1 in, 3 out]
            n514 = Equal?(x=w1093, y=w1098) -> (x = y?=w1094:bool)
            n515 = Equal?(x=w1092, y=w1099) -> (x = y?=w1095:bool)
            n516 = Equal?(x=w1091, y=w1100) -> (x = y?=w1096:bool)
            n517 = Equal?(x=w1090, y=w1101) -> (x = y?=w1097:bool)
            n518 = case shown="False" w1094 {
              frame False {
              }
              frame True {
                n519 = local write "LED 2 STATUS"(FALSE ("LED 1 STATUS")) -> ()
              }
            }
            n520 = case shown="False" w1095 {
              frame False {
              }
              frame True {
                n521 = local write "LED 2 STATUS"(TRUE ("LED 1 STATUS")) -> ()
              }
            }
            n522 = case shown="False" w1096 {
              frame False {
              }
              frame True {
                n523 = local write "LED 1 STATUS"(FALSE ("LED 1 STATUS")) -> ()
              }
            }
            n524 = case shown="False" w1097 {
              frame False {
              }
              frame True {
                n525 = local write "LED 1 STATUS"(TRUE ("LED 1 STATUS")) -> ()
              }
            }
          }
          frame #3 {
            n526 = stacked-sequence {
              frame #0 {
              }
            }
          }
        }
        n527 = local read "SHUTDOWN\nPROGRAM"() -> (w1065:bool)
        "Numeric 4" <- w1064
      }
    }
  }
  n528 = while {
    shift-right: ["Tab Control"] -> _
    shift-left: _ -> [w1108]
    i -> [w1106]
    stop <- w1107 stop-if-true
    n529 = Equal?(x=w1108, y="Tab Control") -> (x = y?=w1110:bool)
    n530 = Wait (ms)(milliseconds to wait=u32 500) -> ()  [unwired: 1 out]
    n531 = local read "SHUTDOWN\nPROGRAM"() -> (w1107:bool)
    n532 = local write "Camera STOP 2"(w1110) -> ()
    "Numeric 5" <- w1106
  }
  n533 = local write "Tab Control"(w5) -> ()
  n534 = while {
    shift-right: [w1115] -> _
    shift-left: w5 -> [w1114]
    i -> [w1113]
    stop <- w1112 stop-if-true
    n535 = case shown="False" "START CAM TAB" {
      tunnel: [w1118 w1119] -> w1115
      tunnel: w1114 -> [_ w1119]
      frame False {
        n536 = local read "Tab Control"() -> (w1118:enum32{"Visible", "Fluorescence"})
      }
      frame True {
      }
    }
    n537 = case shown="\"Fluorescence\"" w1115 {
      frame "Fluorescence" {
        w1125 = errorcluster {"status"=FALSE, "code"=0, "source"=""} ("error in")
        n538 = call "IMAQ Create"("Image Name"="Fluorescence Cam", "error in (no error)"=w1125) -> ("New Image"=w1131:T7)  [unwired: 3 in, 1 out]
        n539 = call <vilib>:"IMAQdx Open Camera.vi"("error in"=w1125, "Session In"="Session In 2") -> ("error out"=w1127:errorcluster, "Session Out"=w1128:T2)  [unwired: 8 in]
        n540 = call <vilib>:"IMAQdx Configure Grab.vi"("error in"=w1127, "Session In"=w1128) -> ("error out"=w1130:errorcluster, "Session Out"=w1129:T2)  [unwired: 8 in]
        n541 = while {
          shift-right: [w1141] -> w1120
          shift-left: w1129 -> [w1143]
          shift-right: [w1140] -> w1121
          shift-left: w1130 -> [w1142]
          shift-right: [w1139] -> _
          shift-left: w1131 -> [w1139]
          i -> [w1137]
          stop <- w1136 continue-if-true
          n542 = call <vilib>:"IMAQdx Grab2.vi"("error in"=w1142, "Image In"=w1139, "Session In"=w1143) -> ("error out"=w1140:errorcluster, "Image Out"=→"Fluorescence Image":T7, "Session Out"=w1141:T2)  [unwired: 5 in, 1 out]
          n543 = Wait (ms)(milliseconds to wait=u32 10) -> ()  [unwired: 1 out]
          n544 = local read "Camera STOP 2"() -> (w1136:bool)
          n545 = local write "START CAM TAB"(w1136) -> ()
          "Numeric" <- w1137
        }
        n546 = Equal?(x=T2 refnum ("Session Out"), y=w1120) -> (x = y?=w1122:bool)
        n547 = case shown="False" w1122 {
          tunnel: w1120 -> [w1133 w1135]
          tunnel: w1121 -> [w1132 w1134]
          frame False {
            n548 = call <vilib>:"IMAQdx Close Camera.vi"("error in"=w1132, "Session In"=w1133) -> ()  [unwired: 9 in, 1 out]
          }
          frame True {
            n549 = call <vilib>:"IMAQdx Close Camera.vi"("error in"=w1134, "Session In"=w1135) -> ()  [unwired: 9 in, 1 out]
          }
        }
      }
      frame "Visible" {
        w1154 = errorcluster {"status"=FALSE, "code"=0, "source"=""} ("error in")
        n550 = call "IMAQ Create"("Image Name"="Visible Cam", "error in (no error)"=w1154) -> ("New Image"=w1151:T7)  [unwired: 3 in, 1 out]
        n551 = call <vilib>:"IMAQdx Open Camera.vi"("error in"=w1154, "Session In"="Session In") -> ("error out"=w1152:errorcluster, "Session Out"=w1153:T2)  [unwired: 8 in]
        n552 = call <vilib>:"IMAQdx Configure Grab.vi"("error in"=w1152, "Session In"=w1153) -> ("error out"=w1149:errorcluster, "Session Out"=w1150:T2)  [unwired: 8 in]
        n553 = while {
          shift-right: [w1163] -> _
          shift-left: w1151 -> [w1163]
          shift-right: [w1162] -> w1146
          shift-left: w1150 -> [w1165]
          shift-right: [w1161] -> w1148
          shift-left: w1149 -> [w1164]
          i -> [w1160]
          stop <- w1159 continue-if-true
          n554 = Wait (ms)(milliseconds to wait=u32 10) -> ()  [unwired: 1 out]
          n555 = call <vilib>:"IMAQdx Grab2.vi"("error in"=w1164, "Image In"=w1163, "Session In"=w1165) -> ("error out"=w1161:errorcluster, "Image Out"=→"Visible Image":T7, "Session Out"=w1162:T2)  [unwired: 5 in, 1 out]
          n556 = local read "Camera STOP 2"() -> (w1159:bool)
          n557 = local write "START CAM TAB"(w1159) -> ()
          "Numeric 2" <- w1160
        }
        n558 = Equal?(x=T2 refnum ("Session Out"), y=w1146) -> (x = y?=w1145:bool)
        n559 = case shown="True" w1145 {
          tunnel: w1148 -> [w1158 _]
          tunnel: w1146 -> [w1157 _]
          frame False {
            n560 = call <vilib>:"IMAQdx Close Camera.vi"("error in"=w1158, "Session In"=w1157) -> ()  [unwired: 9 in, 1 out]
          }
          frame True {
          }
        }
      }
    }
    n561 = Wait (ms)(milliseconds to wait=u32 10) -> ()  [unwired: 1 out]
    n562 = local read "CAMERA STOP"() -> (w1112:bool)
    "Numeric 6" <- w1113
  }
  n563 = stacked-sequence {
    frame #0 {
      n564 = while {
        stop <- w1170 stop-if-true
        n565 = local read "SHUTDOWN\nPROGRAM"() -> (w1169:bool)
        n566 = local read "ABORT \nLOOP"() -> (w1168:bool)
        n567 = local read "LASER\nOFF"() -> (w1172:bool)
        n568 = Compound Arithmetic op=OR(w1169, w1172, w1168) -> (w1171:bool)
        n569 = case shown="False" w1171 {
          tunnel: [FALSE ("SHUTDOWN\nPROGRAM") w1176] -> w1170
          tunnel: w1169 -> [_ w1175]
          frame False {
            n570 = Wait (ms)(milliseconds to wait=u32 10) -> ()  [unwired: 1 out]
          }
          frame True {
            n571 = stacked-sequence {
              seq-local: [_ _ w1180 _ _ _ _ _] -> [_ _ _ _ w1203 _ _ _]
              seq-local: [_ _ w1179 _ _ _ _ _] -> [_ _ _ _ w1204 _ _ _]
              tunnel: [_ _ _ _ _ _ _ TRUE ("SHUTDOWN\nPROGRAM")] -> w1176
              tunnel: w1175 -> [_ _ _ _ _ _ _ _]
              frame #0 {
                n572 = global write "LPT-GUI-MIC-ver 5c GLOBAL 1.0.vi" "SHUTDOWN\nPROGRAM"(TRUE ("SHUTDOWN\nPROGRAM")) -> ()
              }
              frame #1 {
                n573 = Wait (ms)(milliseconds to wait=u32 1200) -> ()  [unwired: 1 out]
              }
              frame #2 {
                n574 = local read "LQC"() -> (w1181:refnum<visa-resource-name>)
                n575 = call "LPT-LQCommSetPower.vi"("LQComm Resource In"=w1187, "Set Power (mW)"=0.0, "error in"=w1186) -> ("LQComm Resource Out"=w1184:refnum<visa-resource-name>, "error out"=w1185:errorcluster)  [unwired: 2 out]
                n576 = while {
                  tunnel: w1184 -> [w1199]
                  tunnel: w1185 -> [w1198]
                  tunnel: [w1195] -> w1179
                  tunnel: [w1194] -> w1180
                  stop <- w1191 stop-if-true
                  n577 = call "LPT-LQCommGetPower.vi"("error in"=w1198, "LQComm Resource In"=w1199) -> ("error out"=w1194:errorcluster, "NumericValue"=w1193:dbl, "LQComm Resource Out"=w1195:refnum<visa-resource-name>)  [unwired: 1 in]
                  n578 = Wait (ms)(milliseconds to wait=u32 50) -> ()  [unwired: 1 out]
                  n579 = local write "Power Out"(w1193) -> ()
                  n580 = Less?(x=w1193, y=0.5) -> (x < y?=w1191:bool)
                  n581 = local write "Status"("Powering Down Raman Laser" ("STATUS")) -> ()
                }
                n582 = flat-sequence {
                  tunnel: errorcluster {"status"=FALSE, "code"=0, "source"=""} ("error out") -> [w1189]
                  tunnel: [w1189] -> w1186
                  tunnel: w1181 -> [w1188]
                  tunnel: [w1188] -> w1187
                  frame #0 {
                    n583 = local write "INTERACTIVE CONTROLS"(6) -> ()
                  }
                }
              }
              frame #3 {
                n584 = Wait (ms)(milliseconds to wait=u32 6000) -> ()  [unwired: 1 out]
              }
              frame #4 {
                n585 = case shown="True" FALSE {
                  tunnel: w1204 -> [_ w1206]
                  tunnel: w1203 -> [_ w1205]
                  frame False {
                  }
                  frame True {
                    n586 = call "LPT-LQOFF.vi"("error in"=w1205, "LQComm Resource In"=w1206) -> ("error out"=w1207:errorcluster, "LQComm Resource Out"=w1208:refnum<visa-resource-name>)  [unwired: 1 in, 1 out]
                    n587 = call "LPT-LQCommClose.vi"("error in (no error)"=w1207, "LQ Resource In"=w1208) -> ()  [unwired: 1 out]
                  }
                }
                n588 = local write "Status"("Closing Application" ("STATUS")) -> ()
              }
              frame #5 {
                n589 = local read "LASER\nOFF"() -> (w1210:bool)
                n590 = case shown="False" w1210 {
                  frame False {
                    n591 = local write "CAMERA STOP"(TRUE ("Camera STOP")) -> ()
                    n592 = local write "START CAM TAB"(FALSE ("START CAM TAB")) -> ()
                    n593 = local write "Camera STOP 2"(FALSE ("Camera STOP 2")) -> ()
                  }
                  frame True {
                  }
                }
                n594 = local write "LASER\nOFF"(FALSE ("LASER\nOFF")) -> ()
                n595 = local write "Start"(FALSE) -> ()
              }
              frame #6 {
                n596 = Wait (ms)(milliseconds to wait=u32 10) -> ()  [unwired: 1 out]
              }
              frame #7 {
                n597 = local write "Status"("Application closed") -> ()
                n598 = property on="SHUTDOWN\nPROGRAM" class="Bool (strict)"("Strings [4]"=string[] ["SHUTDOWN\nPROGRAM", "SHUTDOWN\nPROGRAM", "SHUTDOWN\nPROGRAM", "SHUTDOWN\nPROGRAM"] ("output array")) -> ()  [unwired: 2 in, 2 out]
              }
            }
          }
        }
      }
    }
  }
  "LASER \nFOCUSED" <- FALSE ("Laser \nFocused")
  "Camera STOP 2" <- TRUE ("Camera STOP 2")
